vi "Location Defaults.vi"(0 "Motion Settings In":T22={"No Motion?"=FALSE, "Motion System"=enum."NI 735x", "Motion Bd ID"=1, "Motion Profile"="SMAC1", "# Axis"=1, "Reverse Z axis?"=TRUE, "SMAC Axis"=0, "scan pair"=enum."y-(x) scan", "RT fps"=6.0, "Steps per mm"=[1000, 1000, 1000, 1000], "Motor Parameters"={"velocity ct/s"=[10000.0, 10000.0, 10000.0, 50000.0], "accel ct/s^2"=[50000.0, 50000.0, 50000.0, 200000.0]}, "One Way Scan"=FALSE, "Reverse One Way Scan"=FALSE, "Global Position (mm)"=[], "Plane"=0, "Distance between\nscan lines (um)"=0.0, "Distance between\nscan planes (um)"=0.0, "number of scan planes"=1, "Total steps in line"=0, "Xtra plane\ndistance  (um)"=100, "Xtra planes "=1, "Add Axis"=FALSE, "overshoot cts"=200, "BKPT Shift"=0, "Scan Start Time (ms)"=0, "ESP VISA"="GPIB::1::INSTR", "3rd Axis"=1, "GL Ref Out"=refnum, "Galil Address"=""} {"3rd Axis" items=["x", "y", "z", "w"]; "Xtra planes" min=1; "Xtra plane\ndistance  (um)" min=0; "Distance between\nscan planes (um)" format="%.2f"; "Distance between\nscan lines (um)" format="%.2f"; "SMAC Axis" items=["None"=0, "Axis 1"=1, "Axis 2"=2, "Axis 3"=3, "Axis 4"=4, "Axis 5"=5, "Axis 6"=6, "Axis 7"=7, "Axis 8"=8, "Vector Space 1"=17, "Vector Space 2"=18, "Vector Space 3"=19, "Vector Space 4"=20]; "Motion Bd ID" min=1 max=32 step=1}, 1 "Motion System":T1=enum."No Motion Card", 2 "Debug Mode?":bool, 5 "Digitizer Settings In":T25={"Digitizer delay (us) "=0.0, "rf points per line"=2048, "lines per plane"=128, "Samp Rate (Hz)"=100000000.0, "Additional dig delay (us)"=0.0, "Voltage Scale"=0.4, "Pre-Looks"=0, "Offset delay (us)"=0.0, "bits A/D"=8, "Avg Num"=1, "DigTimeOut"=5.0, "Rel Dig Delay"=0.0, "Dig Ch"=0, "LeCroyCluster"={"LeCroy Channels"=[TRUE, FALSE, FALSE, FALSE], "LC read pt offset"=0.0, "Sweep Avg"=FALSE}, "Main Digitizer"=enum."NI Digitizer", "Dig Config"=enum."Single channel", "Digitizer ID Cluster"={"Acqiris/Alazar/SP ID"=[], "NI Instr Handles"=[], "LeCroy VISA"="", "GaGe Handle"={"Handle"=0, "Sample size"=0, "Resolution"=0, "Offset"=0, "Channels"=0, "Boards"=0}, "ATS Ref"="ATS9350", "Acqiris Address"=["PCI::INSTR0"], "ADQRef"=refnum, "adq_cu_ptr"=refnum}, "Trigger Settings"={"Trig Source"=1, "Trig Coupling"=0, "Trig Slope"=0, "Level (mV)"=1500.0}, "Bulk Acq"=FALSE, "Bulk Start Indexes"=[], "Data Ref RF"=refnum, "NI ID/Channel"=[], "Total Dig CH"=1, "Xtra Ann Trig delay (us)"=10.0, "Fix Z Delay?"=FALSE, "One Way Transmission?"=FALSE, "Data Ref Log"=refnum} {"Trigger Settings"."Trig Slope" items=["Positive", "Negative"]; "Trigger Settings"."Level (mV)" format="%.2f"; "Trigger Settings"."Trig Coupling" items=["DC 1 MOhm", "AC 1 MOhm", "DC 50 Ohm", "AC 50 Ohm"]; "Trigger Settings"."Trig Source" items=["Chan 1", "External"]; "Rel Dig Delay" format="%.2f"; "DigTimeOut" format="%.2f"; "Avg Num" min=1; "Offset delay (us)" format="%.2f"; "Additional dig delay (us)" format="%.2f"; "Digitizer delay (us)" format="%.2f"}, 6 "LeCroy IP Address":refnum<visa-resource-name>="USB0::0x05FF::0x1023::3561N17635::INSTR", 7 "Microscopy Scope":refnum<visa-resource-name>="HDO6104", 9 "Location In":T30=enum."WCM Main", 11 "Computer Name":string, 12 "Create Data Folder":bool) -> (3 "Bypass 2nd dig init":bool, 4 "Motion Settings":T22={"No Motion?"=FALSE, "Motion System"=enum."MM3000", "Motion Bd ID"=0, "Motion Profile"="SMAC1", "# Axis"=0, "Reverse Z axis?"=FALSE, "SMAC Axis"=0, "scan pair"=enum."y-(x) scan", "RT fps"=0.0, "Steps per mm"=[], "Motor Parameters"={"velocity ct/s"=[], "accel ct/s^2"=[]}, "One Way Scan"=FALSE, "Reverse One Way Scan"=FALSE, "Global Position (mm)"=[], "Plane"=0, "Distance between\nscan lines (um)"=0.0, "Distance between\nscan planes (um)"=0.0, "number of scan planes"=0, "Total steps in line"=0, "Xtra plane\ndistance  (um)"=0, "Xtra planes "=0, "Add Axis"=FALSE, "overshoot cts"=0, "BKPT Shift"=0, "Scan Start Time (ms)"=0, "ESP VISA"="", "3rd Axis"=1, "GL Ref Out"=refnum, "Galil Address"=""} {"3rd Axis" items=["x", "y", "z", "w"]; "Xtra planes" min=1; "Xtra plane\ndistance  (um)" min=0; "Distance between\nscan planes (um)" format="%.2f"; "Distance between\nscan lines (um)" format="%.2f"; "SMAC Axis" items=["None"=0, "Axis 1"=1, "Axis 2"=2, "Axis 3"=3, "Axis 4"=4, "Axis 5"=5, "Axis 6"=6, "Axis 7"=7, "Axis 8"=8, "Vector Space 1"=17, "Vector Space 2"=18, "Vector Space 3"=19, "Vector Space 4"=20]; "Motion Bd ID" min=1 max=32 step=1}, 8 "Digitizer Settings":T25={"Digitizer delay (us) "=0.0, "rf points per line"=2048, "lines per plane"=128, "Samp Rate (Hz)"=100000000.0, "Additional dig delay (us)"=0.0, "Voltage Scale"=0.4, "Pre-Looks"=0, "Offset delay (us)"=0.0, "bits A/D"=8, "Avg Num"=1, "DigTimeOut"=5.0, "Rel Dig Delay"=0.0, "Dig Ch"=0, "LeCroyCluster"={"LeCroy Channels"=[TRUE, FALSE, FALSE, FALSE], "LC read pt offset"=0.0, "Sweep Avg"=FALSE}, "Main Digitizer"=enum."NI Digitizer", "Dig Config"=enum."Single channel", "Digitizer ID Cluster"={"Acqiris/Alazar/SP ID"=[], "NI Instr Handles"=[], "LeCroy VISA"="", "GaGe Handle"={"Handle"=0, "Sample size"=0, "Resolution"=0, "Offset"=0, "Channels"=0, "Boards"=0}, "ATS Ref"="ATS9350", "Acqiris Address"=["PCI::INSTR0"], "ADQRef"=refnum, "adq_cu_ptr"=refnum}, "Trigger Settings"={"Trig Source"=1, "Trig Coupling"=0, "Trig Slope"=0, "Level (mV)"=1500.0}, "Bulk Acq"=FALSE, "Bulk Start Indexes"=[], "Data Ref RF"=refnum, "NI ID/Channel"=[], "Total Dig CH"=1, "Xtra Ann Trig delay (us)"=10.0, "Fix Z Delay?"=FALSE, "One Way Transmission?"=FALSE, "Data Ref Log"=refnum} {"Trigger Settings"."Trig Slope" items=["Positive", "Negative"]; "Trigger Settings"."Level (mV)" format="%.2f"; "Trigger Settings"."Trig Coupling" items=["DC 1 MOhm", "AC 1 MOhm", "DC 50 Ohm", "AC 50 Ohm"]; "Trigger Settings"."Trig Source" items=["Chan 1", "External"]; "Rel Dig Delay" format="%.2f"; "DigTimeOut" format="%.2f"; "Avg Num" min=1; "Offset delay (us)" format="%.2f"; "Additional dig delay (us)" format="%.2f"; "Digitizer delay (us)" format="%.2f"}, 10 "Switch T/R":u32=1, 14 "Dual XDCR Settings":T2 {"XDCR Settings"."UT340 Controls"."Low Pass Filter (MHz)" min=-6 max=60 step=1; "XDCR Settings"."UT340 Controls"."High Pass Filter (MHz)" min=1 max=20 step=1; "XDCR Settings"."UT340 Controls"."Rep Rate (Hz)" min=20 step=1; "XDCR Settings"."UT340 Controls"."Pulse Width (ns)" min=100.0 max=250.0 step=2.0; "XDCR Settings"."UT340 Controls"."Voltage" min=100 max=250 step=2; "XDCR Settings"."UT340 Controls"."PC Gain (dB)" min=2 max=72; "XDCR Settings"."UT340 Controls"."PE Gain (dB)" min=-6 max=60 step=1; "XDCR Settings"."JSR Complete"."JSR Trigger Settings"."PRF (Hz)" items=["100 Hz"=0.1, "200 Hz"=0.2, "400 Hz"=0.4, "600 Hz"=0.6, "800 Hz"=0.8, "1000 Hz"=1.0, "1250 Hz"=1.25, "1500 Hz"=1.5, "1750 Hz"=1.75, "2000 Hz"=2.0, "2500 Hz"=2.5, "3000 Hz"=3.0, "3500 Hz"=3.5, "4000 Hz"=4.0, "4500 Hz"=4.5, "5000 Hz"=5.0]; "XDCR Settings"."JSR Complete"."JSR Trigger Settings"."Trigger Source" items=["Internal", "External"]; "XDCR Settings"."JSR Complete"."JSR Trigger Settings"."External Trigger Limit" items=["No Limit", "5 kHz"]; "XDCR Settings"."JSR Complete"."JSR Receive Settings"."Gain (dB)" min=-13 max=66 step=1; "XDCR Settings"."JSR Complete"."JSR Receive Settings"."Low Pass Filter" items=["5 MHz"=5, "10 MHz"=10, "15 MHz"=15, "22.5 MHz"=22, "35 MHz"=35, "50 MHz"=50]; "XDCR Settings"."JSR Complete"."JSR Receive Settings"."High Pass Filter" items=["DC"=0, "1 MHz"=1000, "2.5 MHz"=2500, "5 MHz"=5000, "7.5 MHz"=7500, "12.5 MHz"=12500]; "XDCR Settings"."JSR Complete"."JSR Receive Settings"."Receiver Mode" items=["Echo", "Through"]; "XDCR Settings"."JSR Complete"."JSR Pulse Settings"."Pulser Voltage (V)" items=["100"=100, "125"=125, "150"=150, "175"=175, "200"=200, "225"=225, "250"=250, "275"=275, "300"=300, "325"=325, "350"=350, "375"=375, "400"=400, "425"=425, "450"=450, "475"=475]; "XDCR Settings"."JSR Complete"."JSR Pulse Settings"."Pulser Impedance" items=["High z", "Low z"]; "XDCR Settings"."JSR Complete"."JSR Pulse Settings"."Pulse Energy Level" items=["0 (Minimum)", "1", "2", "3 (Maximum)"]; "XDCR Settings"."JSR Complete"."JSR Pulse Settings"."Damping" items=["331 Ohms"=331, "198 Ohms"=198, "142 Ohms"=142, "110 Ohms"=110, "92 Ohms"=92, "77 Ohms"=77, "67 Ohms"=67, "59 Ohms"=59, "52 Ohms"=52, "47 Ohms"=47, "43 Ohms"=43, "39 Ohms"=39, "37 Ohms"=37, "34 Ohms"=34, "32 Ohms"=32, "30 Ohms"=30]; "XDCR Settings"."Panametrics Settings"."FINE ATTENUATION" items=["00.0", "00.5", "01.0", "01.5", "02.0", "02.5", "03.0", "03.5", "04.0", "04.5", "05.0", "05.5", "06.0", "06.5", "07.0", "07.5", "08.0", "08.5", "09.0", "09.5", "10.0", "10.5", "11.0", "11.5", "12.0", "12.5", "13.0", "13.5", "14.0", "14.5", "15.0", "15.5"]; "XDCR Settings"."Panametrics Settings"."COARSE ATTENUATION" items=["00.0", "10.0", "20.0", "30.0", "40.0", "50.0"]; "XDCR Settings"."Panametrics Settings"."GAIN (db)" items=["26.0", "40.0", "54.0"]; "XDCR Settings"."Panametrics Settings"."PRF (KHz)" items=["XREMT", "EXBNC", "0.200", "0.500", "1.000", "2.000", "5.000", "10.00", "20.00"]; "XDCR Settings"."Panametrics Settings"."MODE" items=["P/ E", "THRU", "RPP", "EXT_PLSR"]; "XDCR Settings"."Panametrics Settings"."LP FILT (MHz)" items=["20", "50", "100", "200"]; "XDCR Settings"."Panametrics Settings"."HP FILT (KHz)" items=["1", "1000", "3000", "10000"]; "XDCR Settings"."Panametrics Settings"."DAMPING (Ohm)" items=["7", "10", "16", "20", "26", "30", "40", "50"]; "XDCR Settings"."Panametrics Settings"."ENERGY (uJ)" items=["1", "2", "4", "8", "16", "32"]; "XDCR Settings"."Daxsonics Settings"."Freq (MHz)" items=["4"=4, "5"=5, "6"=6, "8"=8, "10"=10, "12"=12, "14"=14, "15"=15, "16"=16, "17"=17, "18"=18, "20"=20, "25"=25, "30"=30, "35"=35, "40"=40, "45"=45, "50"=50]; "XDCR Settings"."Daxsonics Settings"."Voltage (V)" items=["0"=0, "5"=5, "10"=10, "15"=15, "20"=20, "25"=25, "30"=30, "35"=35, "40"=40, "45"=45, "50"=50, "55"=55, "60"=60, "65"=65, "70"=70, "75"=75, "80"=80, "85"=85, "90"=90, "95"=95, "100"=100, "110"=110, "120"=120, "130"=130, "140"=140, "150"=150, "160"=160, "170"=170, "180"=180, "190"=190]; "XDCR Settings"."Daxsonics Settings"."Gain (dB)" items=["22"=22, "25"=25, "28"=28, "31"=31, "34"=34, "37"=37, "40"=40, "43"=43, "46"=46, "49"=49, "52"=52, "55"=55, "58"=58, "61"=61, "64"=64, "67"=67]; "XDCR Settings"."Digitizer Settings"."Additional dig delay (ms)" format="%.2f"; "XDCR Settings"."Digitizer Settings"."Time scale per Div" items=["100 ns"=0.1, "200 ns"=0.2, "500 ns"=0.5, "1 micros"=1.0, "2 micros"=2.0, "5 micros"=5.0, "10 micros"=10.0, "20 micros"=20.0, "50 micros"=50.0, "100 micros"=100.0, "200 micros"=200.0, "500 micros"=500.0, "1 ms"=1000.0, "2 ms"=2000.0, "5 ms"=5000.0, "10 ms"=10000.0, "20 ms"=20000.0, "50 ms"=50000.0, "100 ms"=100000.0, "200 ms"=200000.0]; "XDCR Settings"."Digitizer Settings"."RF data Sampling"."rf points per line" min=1; "XDCR Settings"."Digitizer Settings"."RF data Sampling"."Ref Delay (ms)" format="%.2f"}, 15 "Hardware Addresses":T29)   [LabVIEW 2022 SP3]
uses:
  Motion Controllers/NI_controller/-NI_MotionRoutines/MotionParameters.ctl
  Motion Controllers/NI_controller/-NI_MotionRoutines/MotionSys.ctl
  Motion Controllers/-MotionRoutines/ScanAxis.ctl
  Motion Controllers/-MotionRoutines/3rdAxis.ctl
  -ScanSystem/Controls/location.ctl
  Digitizers/-DigitizerRoutines/DigitizerSettings.ctl
  Digitizers/-DigitizerRoutines/Digitizer.ctl
  Digitizers/-DigitizerRoutines/DigConfig.ctl
  Digitizers/-DigitizerRoutines/DigitizerID.ctl
  C:/Windows/System32/ADQAPI_dotNet_helper.dll
  Windows/System32/ADQAPI_dotNet_helper.dll
  DualXDCR/Dual XDCR Complete Settings.ctl
  DualXDCR/XDCRSettings.ctl
  Pulsers/Daxsonics/-DaxSubroutines/Dax_Control_Cluster.ctl
  Pulsers/Panametrics/Pana5900.ctl
  Pulsers/JSR/Controls/JSR Complete.ctl
  Pulsers/JSR/Controls/JSR Pulse.ctl
  Pulsers/JSR/Controls/Damping.ctl
  Pulsers/JSR/Controls/Energy.ctl
  Pulsers/JSR/Controls/Z.ctl
  Pulsers/JSR/Controls/Volt.ctl
  Pulsers/JSR/Controls/JSR Recieve.ctl
  Pulsers/JSR/Controls/Mode.ctl
  Pulsers/JSR/Controls/HPF.ctl
  Pulsers/JSR/Controls/LPF.ctl
  Pulsers/JSR/Controls/Gain.ctl
  Pulsers/JSR/Controls/JSR Trigger.ctl
  Pulsers/JSR/Controls/Trig Limit.ctl
  Pulsers/JSR/Controls/Trig Source.ctl
  Pulsers/JSR/Controls/PRF.ctl
  Pulsers/UTEX/Controls/UTEX Controls.ctl
  Motion Controllers/-MotionRoutines/MotionGlobals.vi
  Pulsers/PulserGlobals.vi
  Switch Modules/SwitchGlobals.vi
panel:
  in  "Microscopy Scope 2":refnum<visa-resource-name>="HDO6104"
  # "1-D and 2-D B scan settings"
  # "1-D and 2-D B scan settings"
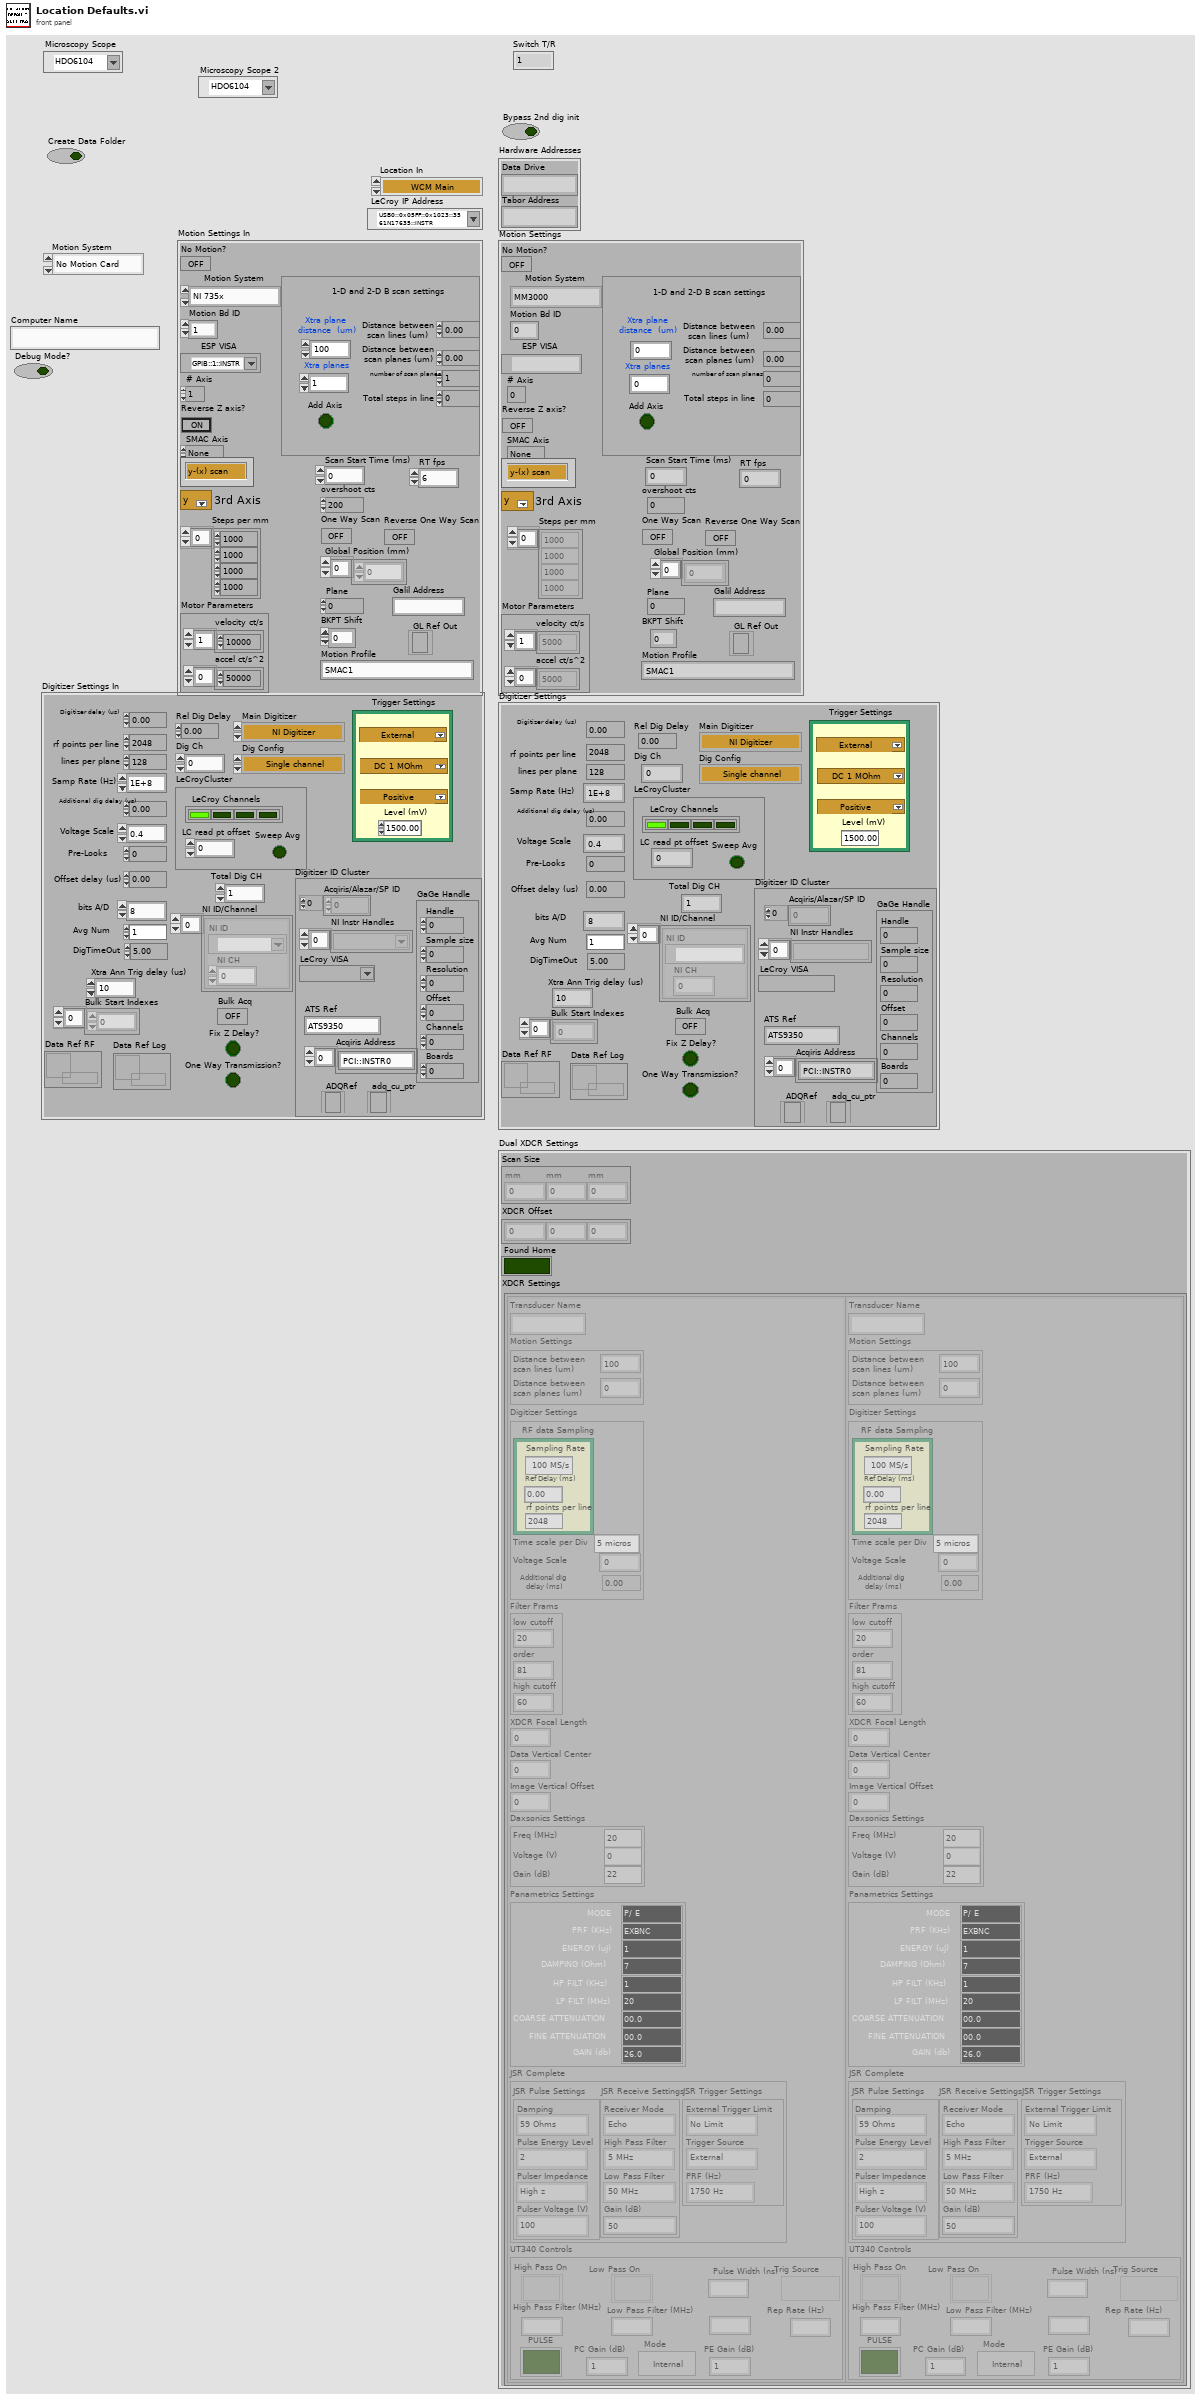
[diagram p1: front panel]
types:
  T1 = typedef "MotionSys.ctl" = enum16{"MM3000", "NI 735x", "Newport ESP", "No Motion Card", "Galil"}
  T2 = typedef "Dual XDCR Complete Settings.ctl" = cluster{"Scan Size":dbl[], "XDCR Offset":dbl[], "Found Home":bool, "XDCR Settings":T3[]}
  T3 = typedef "XDCRSettings.ctl" = cluster{"Transducer Name":string, "Motion Settings":cluster{"Distance between\nscan lines (um)":sgl, "Distance between\nscan planes (um)":sgl}, "Digitizer Settings":cluster{"RF data Sampling":cluster{"Sampling Rate":dbl, "Ref Delay (ms)":dbl, "rf points per line":i32}, "Time scale per Div":dbl, "Voltage Scale":dbl, "Additional dig delay (ms)":dbl}, "Filter Prams":cluster{"low cutoff":i32, "order":i32, "high cutoff":i32}, "XDCR Focal Length":dbl, "Data Vertical Center":dbl, "Image Vertical Offset":dbl, "Daxsonics Settings":T4, "Panametrics Settings":T5, "JSR Complete":T6, "UT340 Controls":T21}
  T4 = typedef "Dax_Control_Cluster.ctl" = cluster{"Freq (MHz) ":u16, "Voltage (V)":u16, "Gain (dB)":u16}
  T5 = typedef "Pana5900.ctl" = cluster{"ENERGY (uJ)":u16, "DAMPING (Ohm)":u16, "HP FILT (KHz) ":u16, "LP FILT (MHz)":u16, "MODE":u16, "PRF (KHz)":u16, "GAIN (db)":u16, "COARSE ATTENUATION":u16, "FINE ATTENUATION":u16}
  T6 = typedef "JSR Complete.ctl" = cluster{"JSR Pulse Settings":T7, "JSR Receive Settings":T12, "JSR Trigger Settings":T17}
  T7 = typedef "JSR Pulse.ctl" = cluster{"Damping":T8, "Pulse Energy Level":T9, "Pulser Impedance":T10, "Pulser Voltage (V)":T11}
  T8 = typedef "Damping.ctl" = i16
  T9 = typedef "Energy.ctl" = u16
  T10 = typedef "Z.ctl" = u16
  T11 = typedef "Volt.ctl" = i16
  T12 = typedef "JSR Recieve.ctl" = cluster{"Receiver Mode":T13, "High Pass Filter":T14, "Low Pass Filter":T15, "Gain (dB)":T16}
  T13 = typedef "Mode.ctl" = i8
  T14 = typedef "HPF.ctl" = u16
  T15 = typedef "LPF.ctl" = u16
  T16 = typedef "Gain.ctl" = i8
  T17 = typedef "JSR Trigger.ctl" = cluster{"External Trigger Limit":T18, "Trigger Source":T19, "PRF (Hz)":T20}
  T18 = typedef "Trig Limit.ctl" = i8
  T19 = typedef "Trig Source.ctl" = i8
  T20 = typedef "PRF.ctl" = dbl
  T21 = typedef "UTEX Controls.ctl" = cluster{"High Pass On":bool, "High Pass Filter (MHz)":i16, "Low Pass On":bool, "Low Pass Filter (MHz)":i16, "PE Gain (dB)":i16, "Voltage":i16, "Pulse Width (ns)":dbl, "Mode":bool, "PC Gain (dB)":i16, "Trig Source":bool, "Rep Rate (Hz)":i16, "PULSE":bool}
  T22 = typedef "MotionParameters.ctl" = cluster{"No Motion?":bool, "Motion System":T1, "Motion Bd ID":u8, "Motion Profile":string, "# Axis":i8, "Reverse Z axis?":bool, "SMAC Axis":u16, "scan pair":T23, "RT fps":sgl, "Steps per mm":i32[], "Motor Parameters":cluster{"velocity ct/s":dbl[], "accel ct/s^2":dbl[]}, "One Way Scan":bool, "Reverse One Way Scan":bool, "Global Position (mm)":dbl[], "Plane":i32, "Distance between\nscan lines (um)":sgl, "Distance between\nscan planes (um)":sgl, "number of scan planes":i32, "Total steps in line":i32, "Xtra plane\ndistance  (um)":i32, "Xtra planes ":i32, "Add Axis":bool, "overshoot cts":i32, "BKPT Shift":i32, "Scan Start Time (ms)":u32, "ESP VISA":refnum<visa-resource-name>, "3rd Axis":T24, "GL Ref Out":refnum<k7>, "Galil Address":string}
  T23 = typedef "ScanAxis.ctl" = enum16{"y-(x) scan", "x-(y) scan", "z-(x) scan", "z-(y) scan", "y-(z) scan", "x-(z) scan", "w-(x) scan", "w-(y) scan", "w-(z) scan", "x-(w) scan", "y-(w) scan", "z-(w) scan"}
  T24 = typedef "3rdAxis.ctl" = u16
  T25 = typedef "DigitizerSettings.ctl" = cluster{"Digitizer delay (us) ":dbl, "rf points per line":i32, "lines per plane":i32, "Samp Rate (Hz)":dbl, "Additional dig delay (us)":dbl, "Voltage Scale":dbl, "Pre-Looks":i32, "Offset delay (us)":dbl, "bits A/D":i8, "Avg Num":i32, "DigTimeOut":sgl, "Rel Dig Delay":sgl, "Dig Ch":i32, "LeCroyCluster":cluster{"LeCroy Channels":bool[], "LC read pt offset":dbl, "Sweep Avg":bool}, "Main Digitizer":T26, "Dig Config":T27, "Digitizer ID Cluster":T28, "Trigger Settings":cluster{"Trig Source":u16, "Trig Coupling":u16, "Trig Slope":u16, "Level (mV)":dbl}, "Bulk Acq":bool, "Bulk Start Indexes":i32[], "Data Ref RF":refnum<data-value>, "NI ID/Channel":cluster{"NI ID":refnum<k15>, "NI CH":i32}[], "Total Dig CH":i32, "Xtra Ann Trig delay (us)":dbl, "Fix Z Delay?":bool, "One Way Transmission?":bool, "Data Ref Log":refnum<data-value>}
  T26 = typedef "Digitizer.ctl" = enum16{"Acqiris Digitizer", "NI Digitizer", "LeCroy", "GaGe", "AlazarTech", "No Digitizer", "Teledyne"}
  T27 = typedef "DigConfig.ctl" = enum16{"Single channel", "2 Chans w/ 2 Acqiris", "2 Chans w/ 1 Acqiris", "5-CH Pulser New", "5-CH pulser w/ ann array", "5-pass style ann array", "Empty"}
  T28 = typedef "DigitizerID.ctl" = cluster{"Acqiris/Alazar/SP ID":u32[], "NI Instr Handles":refnum<k15>[], "LeCroy VISA":refnum<visa-resource-name>, "GaGe Handle":cluster{"Handle":u32, "Sample size":u32, "Resolution":i32, "Offset":i32, "Channels":u32, "Boards":u32}, "ATS Ref":string, "Acqiris Address":string[], "ADQRef":refnum<k24>, "adq_cu_ptr":refnum<k24>}
  T29 = cluster{"Data Drive":string, "Tabor Address":string}
  T30 = typedef "location.ctl" = enum16{"Automatic", "WCM Main", "Hawaii", "Columbia MM3000", "Columbia  NI System", "NYU", "RRI 2", "UHI Allen", "CUMC RT", "Chiba", "Stony Brook", "WCM Microscopy", "WCM Aeoretch", "WCM Optics Lab", "WCM Main 2Axis", "WCM Rotation", "WCM SAM SMAC", "SERI GP", "SERI SAM 2023"}
  T31 = cluster{"velocity mm/s":dbl[], "accel mm/s^2":dbl[]}
  T32 = cluster{"velocity\nmm/s":dbl[], "accel\nmm/s^2":dbl[]}
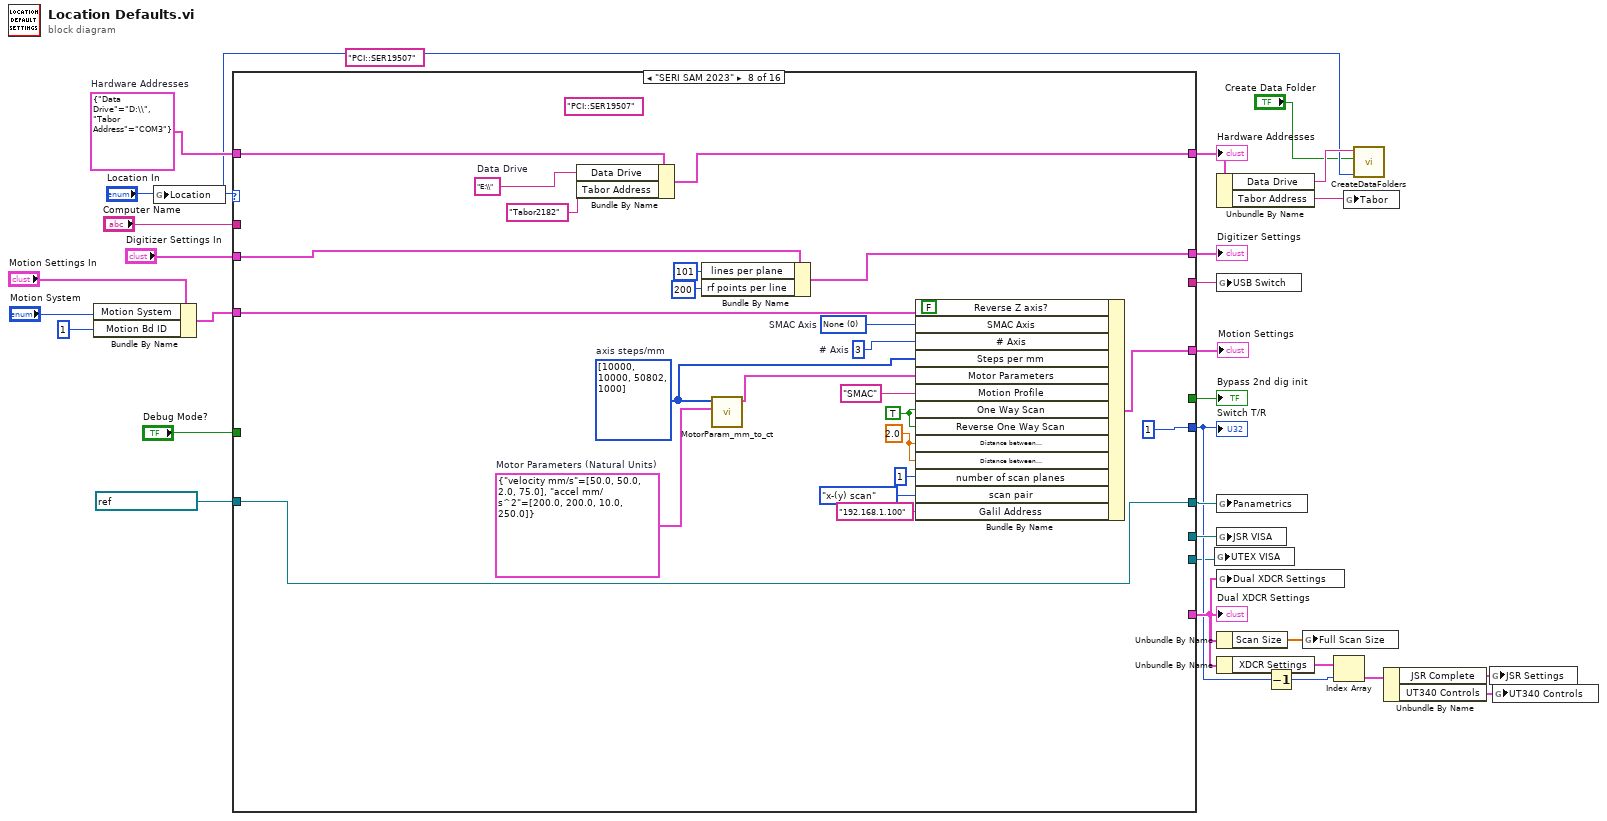
[diagram p0: block diagram]
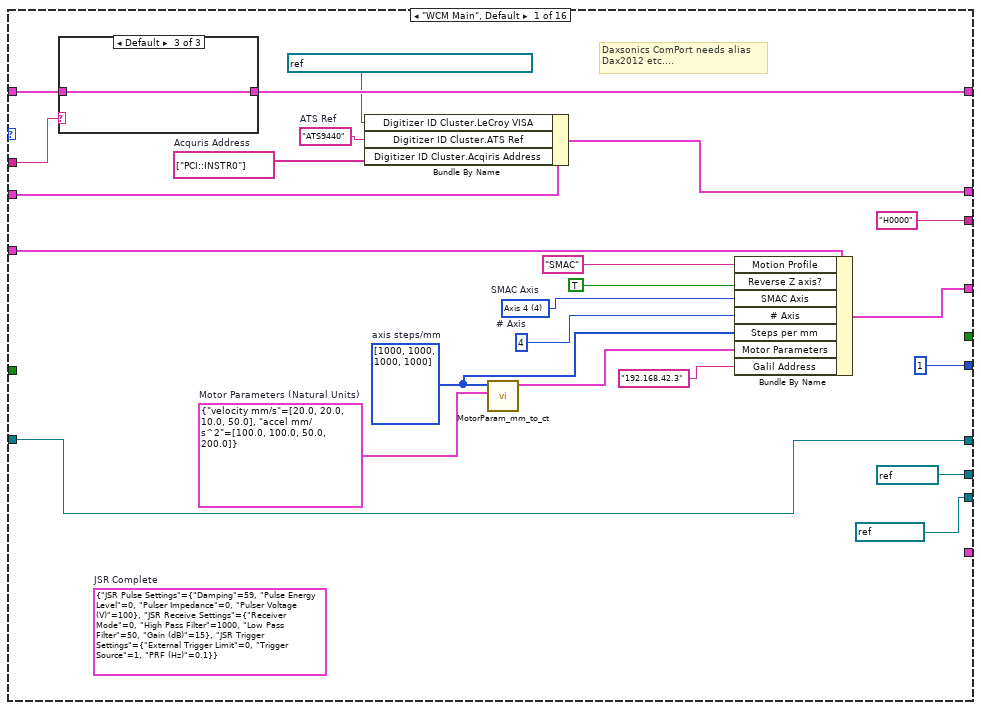
[diagram p2: hidden frame]
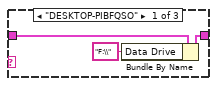
[diagram p3: hidden frame]
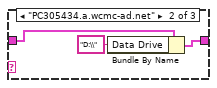
[diagram p4: hidden frame]
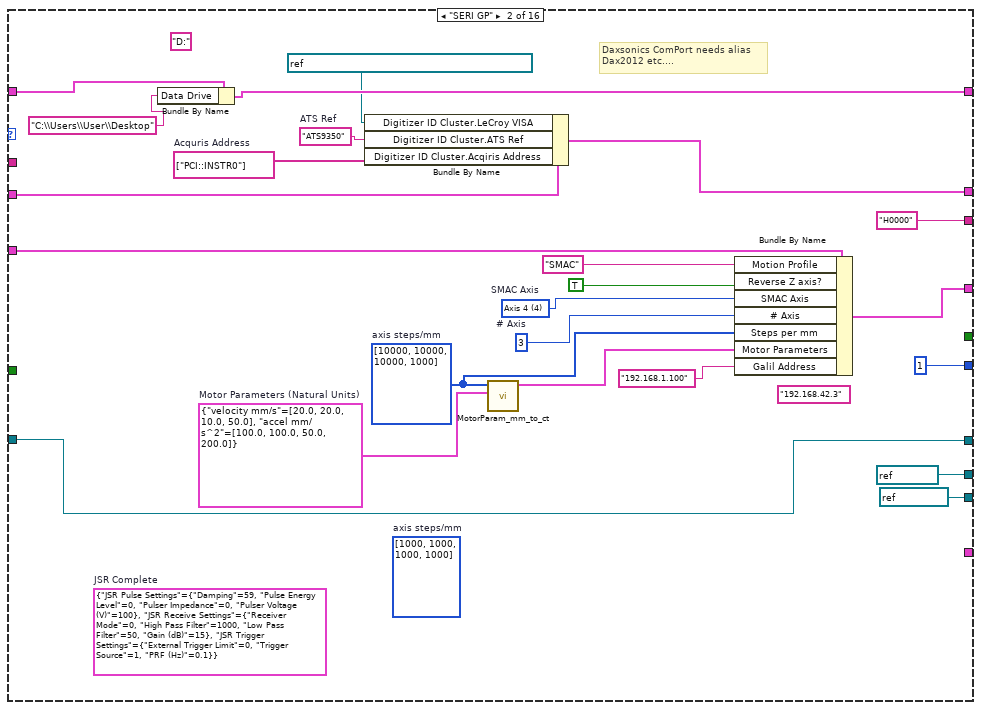
[diagram p5: hidden frame]
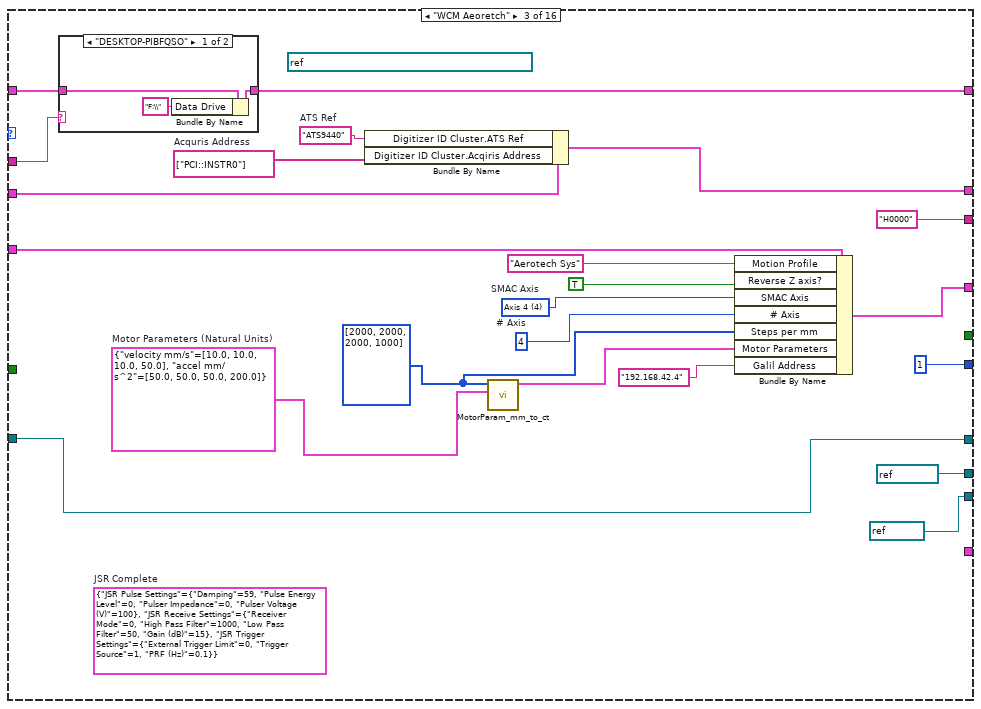
[diagram p6: hidden frame]
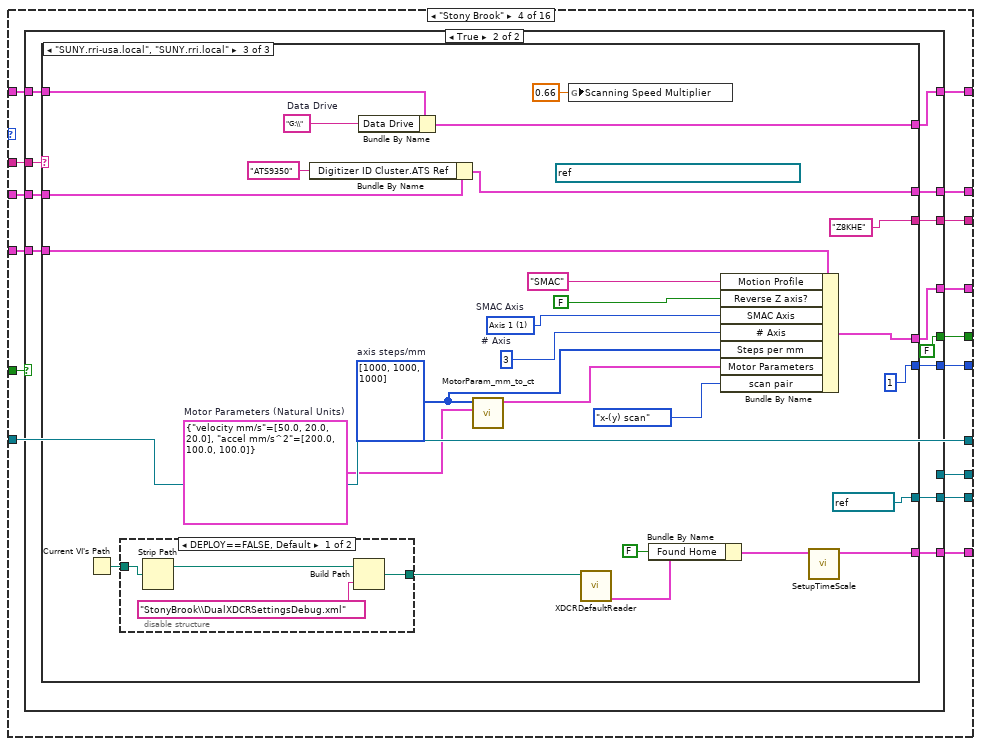
[diagram p8: hidden frame]
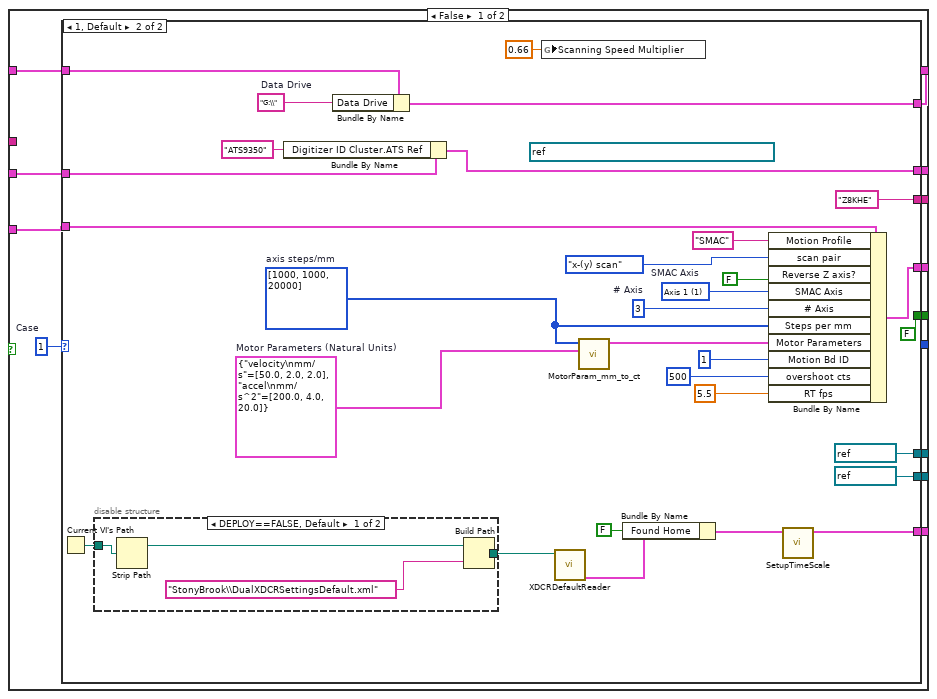
[diagram p9: hidden frame]
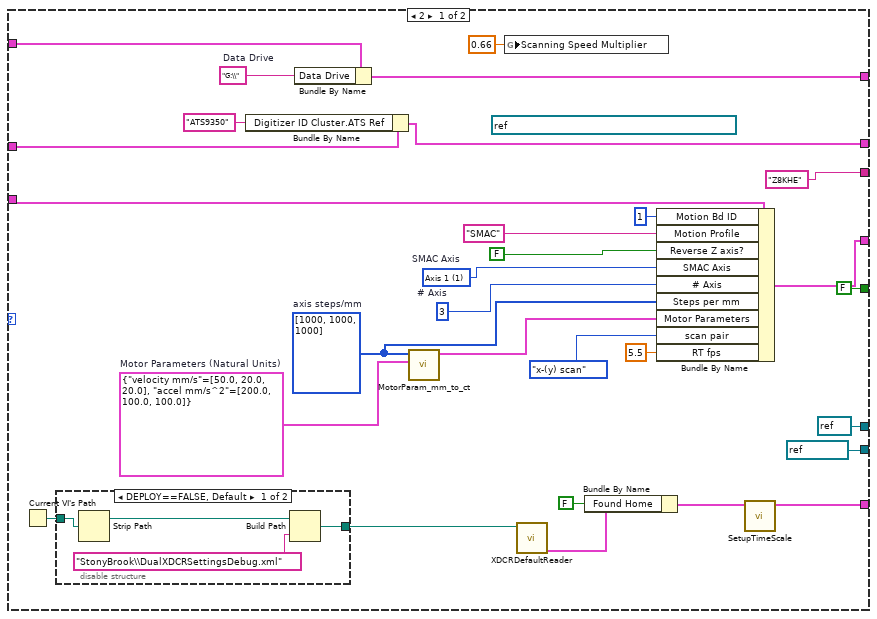
[diagram p10: hidden frame]
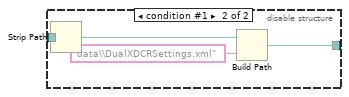
[diagram p11: hidden frame]
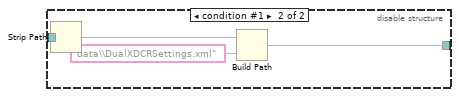
[diagram p12: hidden frame]
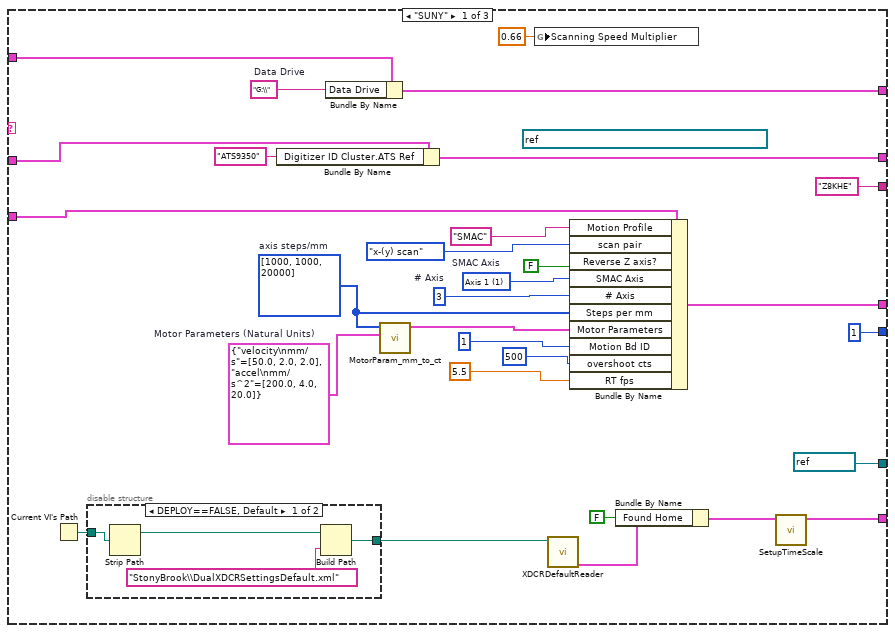
[diagram p13: hidden frame]
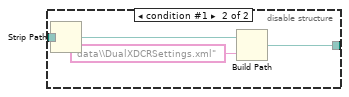
[diagram p14: hidden frame]
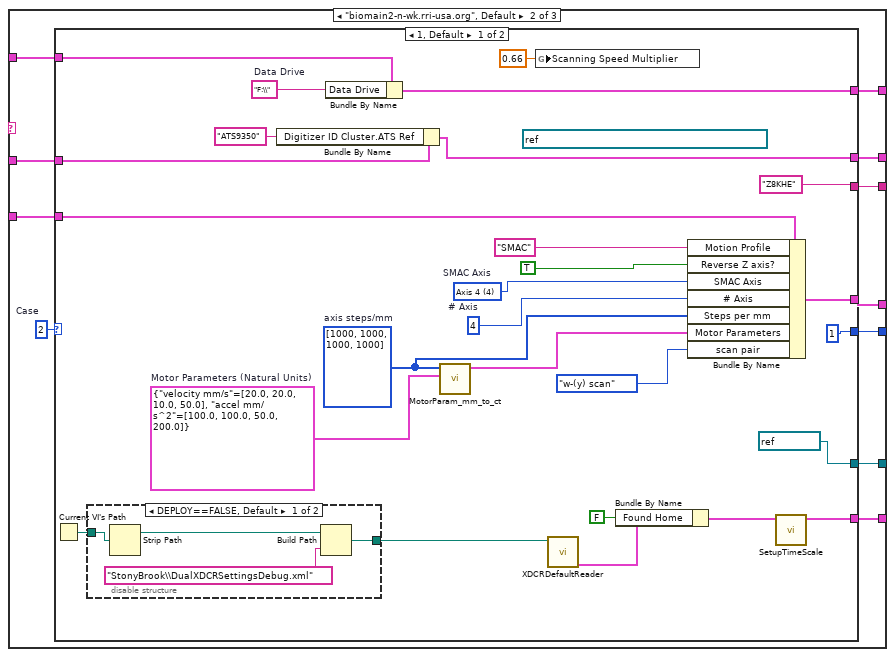
[diagram p15: hidden frame]
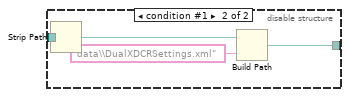
[diagram p16: hidden frame]
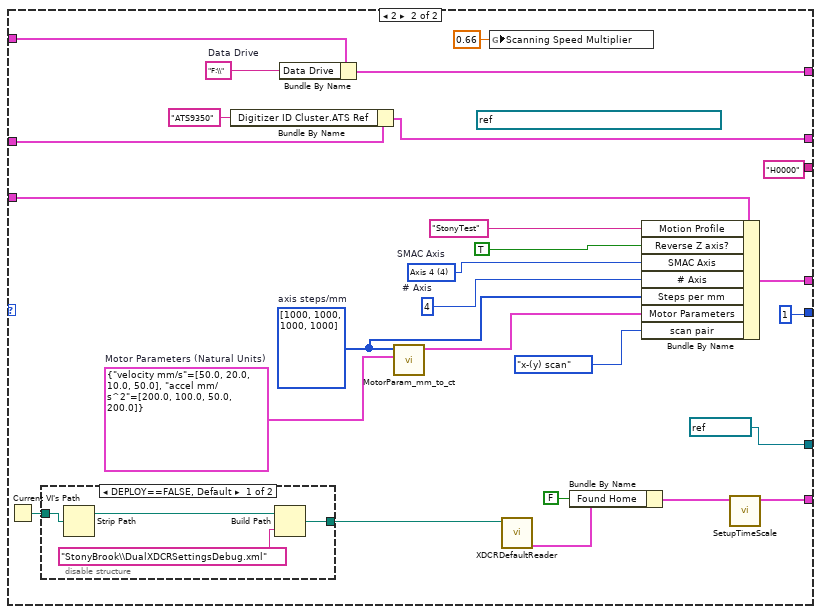
[diagram p17: hidden frame]
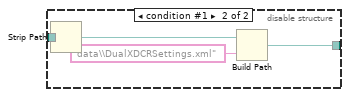
[diagram p18: hidden frame]
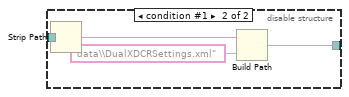
[diagram p19: hidden frame]
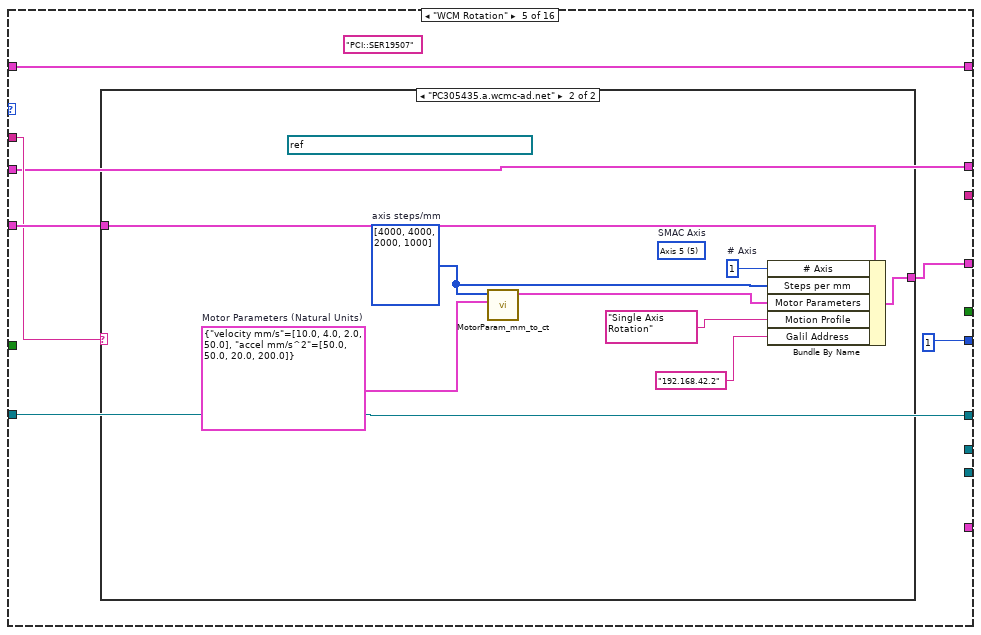
[diagram p20: hidden frame]
diagram:
  (unwired) "PCI::SER19507" ("ResourceName")
  w28 = T29 {"Data Drive"="D:\\", "Tabor Address"="COM3"}  # Hardware Addresses
  n1 = Bundle By Name(cluster="Motion Settings In", "Motion System"="Motion System", "Motion Bd ID"=u8 1 ("Board ID")) -> (w19:T22)
  n2 = global write "MotionGlobals.vi" "Location"("Location In") -> ()
  n3 = case shown="\"SERI SAM 2023\"" "Location In" {
    tunnel: [_ _ _ w118 _ _ _ _ _ _ _ TRUE TRUE _ TRUE _] -> w29
    tunnel: [w52 w82 w104 w123 w379 w418 w442 w466 w476 w490 w498 w655 w675 w700 w716 w738] -> w23
    tunnel: w19 -> [w51 w81 w103 w119 w378 w417 w441 w465 w470 w489 w503 w654 w674 w699 w715 w730]
    tunnel: [w41 w72 w95 w120 w373 w401 w425 w450 w473 w485 w499 w645 w665 w689 w709 w727] -> w22
    tunnel: "Digitizer Settings In" -> [w42 w73 w96 w121 w373 w408 w432 w456 w473 w485 w500 w646 w666 w692 w709 w729]
    tunnel: w28 -> [w38 w69 w92 w122 w377 w411 w435 w459 w472 w483 w502 w650 w670 w693 w711 w731]
    tunnel: [w37 w68 w91 w117 w377 w410 w434 w458 w472 w483 w501 w649 w669 w694 w710 w732] -> w27
    tunnel: [_ _ _ w116 _ _ _ _ _ _ w497 _ _ _ _ _] -> w8
    tunnel: [u32 1 ("Switch T/R") u32 1 ("Switch T/R") u32 1 ("Switch T/R") w109 u32 1 ("Switch T/R") u32 1 ("Switch T/R") u32 1 ("Switch T/R") u32 1 ("Switch T/R") u32 1 ("Switch T/R") u32 1 ("Switch T/R") _ _ _ u32 1 ("Switch T/R") _ _] -> w4
    tunnel: "Computer Name" -> [w36 _ w90 w112 w374 _ _ _ _ _ w493 _ _ _ _ _]
    tunnel: ["H0000" "H0000" "H0000" w115 _ _ _ _ _ _ w496 _ _ _ _ _] -> w14
    tunnel: [w34 w66 w88 w114 w375 w397 w421 w446 w468 w481 w495 refnum<visa-resource-name> "GPIB0::9::INSTR" ("VISA resource name") w658 w680 w708 w725] -> w13
    tunnel: refnum<visa-resource-name> "GPIB::1::INSTR" ("VISA resource name") -> [w34 w66 w88 w114 w375 w397 w421 w446 w468 w481 _ _ w658 w680 w708 w725]
    tunnel: "Debug Mode?" -> [_ _ _ w113 _ _ _ _ _ _ w494 _ _ _ _ _]
    tunnel: [refnum<visa-resource-name> "COM4" ("JSR VISA") refnum<visa-resource-name> "COM4" ("JSR VISA") refnum<visa-resource-name> "COM4" ("JSR VISA") w111 _ _ _ _ _ _ _ _ _ _ _ _] -> w9
    tunnel: [refnum<visa-resource-name> "UTEX" ("JSR VISA") refnum<visa-resource-name> "UTEX" ("JSR VISA") refnum<visa-resource-name> "UTEX" ("JSR VISA") w110 _ _ _ _ _ _ _ _ _ _ _ _] -> w2
    frame "WCM Main", Default {
      (unwired) T6 {"JSR Pulse Settings"={"Damping"=59, "Pulse Energy Level"=0, "Pulser Impedance"=0, "Pulser Voltage (V)"=100}, "JSR Receive Settings"={"Receiver Mode"=0, "High Pass Filter"=1000, "Low Pass Filter"=50, "Gain (dB)"=15}, "JSR Trigger Settings"={"External Trigger Limit"=0, "Trigger Source"=1, "PRF (Hz)"=0.1}}  # JSR Complete
      w40 = "ATS9440"  # ATS Ref
      w39 = string[] ["PCI::INSTR0"]  # Acquris Address
      w47 = i32[] [1000, 1000, 1000, 1000]  # axis steps/mm
      w46 = T31 {"velocity mm/s"=[20.0, 20.0, 10.0, 50.0], "accel mm/s^2"=[100.0, 100.0, 50.0, 200.0]}  # Motor Parameters (Natural Units)
      w48 = i8 4  # # Axis
      w49 = u16 4 items=["None"=0, "Axis 1"=1, "Axis 2"=2, "Axis 3"=3, "Axis 4"=4, "Axis 5"=5, "Axis 6"=6, "Axis 7"=7, "Axis 8"=8, "Vector Space 1"=17, "Vector Space 2"=18, "Vector Space 3"=19, "Vector Space 4"=20]  # SMAC Axis
      # "Daxsonics ComPort needs alias\nDax2012 etc...."
      n4 = case shown="Default" w36 {
        tunnel: w38 -> [w55 w57 w59]
        tunnel: [w54 w56 w59] -> w37
        frame "DESKTOP-PIBFQSO" {
          n5 = Bundle By Name(cluster=w55, "Data Drive"="F:\\") -> (w54:T29)
        }
        frame "PC305434.a.wcmc-ad.net" {
          n6 = Bundle By Name(cluster=w57, "Data Drive"="D:\\") -> (w56:T29)
        }
        frame Default {
        }
      }
      n7 = Bundle By Name(cluster=w42, "Digitizer ID Cluster.LeCroy VISA"=refnum<visa-resource-name> "USB0::0x05FF::0x1023::3504N04910::INSTR" ("VISA resource name"), "Digitizer ID Cluster.ATS Ref"=w40, "Digitizer ID Cluster.Acqiris Address"=w39) -> (w41:T25)
      n8 = call "MotorParam_mm_to_ct.vi"("Motor Parameters (Natural Units)"=w46, "Counts / mm"=w47) -> ("Motoar Parameters (counts)"=w45:cluster{dbl[], dbl[]})  [unwired: 9 in]
      n9 = Bundle By Name(cluster=w51, "Motion Profile"="SMAC", "Reverse Z axis?"=TRUE, "SMAC Axis"=w49, "# Axis"=w48, "Steps per mm"=w47, "Motor Parameters"=w45, "Galil Address"="192.168.42.3" ("For Galil")) -> (w52:T22)
    }
    frame "SERI GP" {
      (unwired) i32[] [1000, 1000, 1000, 1000]  # axis steps/mm
      (unwired) "D:" ("Data Drive")
      (unwired) "192.168.42.3" ("For Galil")
      (unwired) T6 {"JSR Pulse Settings"={"Damping"=59, "Pulse Energy Level"=0, "Pulser Impedance"=0, "Pulser Voltage (V)"=100}, "JSR Receive Settings"={"Receiver Mode"=0, "High Pass Filter"=1000, "Low Pass Filter"=50, "Gain (dB)"=15}, "JSR Trigger Settings"={"External Trigger Limit"=0, "Trigger Source"=1, "PRF (Hz)"=0.1}}  # JSR Complete
      w71 = "ATS9350"  # ATS Ref
      w70 = string[] ["PCI::INSTR0"]  # Acquris Address
      w61 = i32[] [10000, 10000, 10000, 1000]  # axis steps/mm
      w77 = T31 {"velocity mm/s"=[20.0, 20.0, 10.0, 50.0], "accel mm/s^2"=[100.0, 100.0, 50.0, 200.0]}  # Motor Parameters (Natural Units)
      w78 = i8 3  # # Axis
      w79 = u16 4 items=["None"=0, "Axis 1"=1, "Axis 2"=2, "Axis 3"=3, "Axis 4"=4, "Axis 5"=5, "Axis 6"=6, "Axis 7"=7, "Axis 8"=8, "Vector Space 1"=17, "Vector Space 2"=18, "Vector Space 3"=19, "Vector Space 4"=20]  # SMAC Axis
      # "Daxsonics ComPort needs alias\nDax2012 etc...."
      n10 = Bundle By Name(cluster=w69, "Data Drive"="C:\\Users\\User\\Desktop") -> (w68:T29)
      n11 = Bundle By Name(cluster=w73, "Digitizer ID Cluster.LeCroy VISA"=refnum<visa-resource-name> "USB0::0x05FF::0x1023::3504N04910::INSTR" ("VISA resource name"), "Digitizer ID Cluster.ATS Ref"=w71, "Digitizer ID Cluster.Acqiris Address"=w70) -> (w72:T25)
      n12 = call "MotorParam_mm_to_ct.vi"("Motor Parameters (Natural Units)"=w77, "Counts / mm"=w61) -> ("Motoar Parameters (counts)"=w76:cluster{dbl[], dbl[]})  [unwired: 9 in]
      n13 = Bundle By Name(cluster=w81, "Motion Profile"="SMAC", "Reverse Z axis?"=TRUE, "SMAC Axis"=w79, "# Axis"=w78, "Steps per mm"=w61, "Motor Parameters"=w76, "Galil Address"="192.168.1.100" ("For Galil")) -> (w82:T22)
    }
    frame "WCM Aeoretch" {
      w84 = T31 {"velocity mm/s"=[10.0, 10.0, 10.0, 50.0], "accel mm/s^2"=[50.0, 50.0, 50.0, 200.0]}  # Motor Parameters (Natural Units)
      w83 = i32[] [2000, 2000, 2000, 1000]
      (unwired) T6 {"JSR Pulse Settings"={"Damping"=59, "Pulse Energy Level"=0, "Pulser Impedance"=0, "Pulser Voltage (V)"=100}, "JSR Receive Settings"={"Receiver Mode"=0, "High Pass Filter"=1000, "Low Pass Filter"=50, "Gain (dB)"=15}, "JSR Trigger Settings"={"External Trigger Limit"=0, "Trigger Source"=1, "PRF (Hz)"=0.1}}  # JSR Complete
      w94 = "ATS9440"  # ATS Ref
      w93 = string[] ["PCI::INSTR0"]  # Acquris Address
      (unwired) refnum<visa-resource-name> "USB0::0x05FF::0x1023::3504N04910::INSTR" ("VISA resource name")
      w100 = i8 4  # # Axis
      w101 = u16 4 items=["None"=0, "Axis 1"=1, "Axis 2"=2, "Axis 3"=3, "Axis 4"=4, "Axis 5"=5, "Axis 6"=6, "Axis 7"=7, "Axis 8"=8, "Vector Space 1"=17, "Vector Space 2"=18, "Vector Space 3"=19, "Vector Space 4"=20]  # SMAC Axis
      n14 = case shown="\"DESKTOP-PIBFQSO\"" w90 {
        tunnel: w92 -> [w107 w108]
        tunnel: [w106 w108] -> w91
        frame "DESKTOP-PIBFQSO" {
          n15 = Bundle By Name(cluster=w107, "Data Drive"="F:\\") -> (w106:T29)
        }
        frame Default {
        }
      }
      n16 = Bundle By Name(cluster=w96, "Digitizer ID Cluster.ATS Ref"=w94, "Digitizer ID Cluster.Acqiris Address"=w93) -> (w95:T25)
      n17 = call "MotorParam_mm_to_ct.vi"("Motor Parameters (Natural Units)"=w84, "Counts / mm"=w83) -> ("Motoar Parameters (counts)"=w99:cluster{dbl[], dbl[]})  [unwired: 9 in]
      n18 = Bundle By Name(cluster=w103, "Motion Profile"="Aerotech Sys", "Reverse Z axis?"=TRUE, "SMAC Axis"=w101, "# Axis"=w100, "Steps per mm"=w83, "Motor Parameters"=w99, "Galil Address"="192.168.42.4" ("For Galil")) -> (w104:T22)
    }
    frame "Stony Brook" {
      n19 = case shown="True" w113 {
        tunnel: [w135 w218] -> w123
        tunnel: w122 -> [w134 w221]
        tunnel: w121 -> [w133 w215]
        tunnel: [w132 w216] -> w120
        tunnel: w119 -> [w131 w219]
        tunnel: [w130 FALSE] -> w118
        tunnel: [w129 w220] -> w117
        tunnel: [w128 w214] -> w116
        tunnel: [w127 w217] -> w115
        tunnel: w112 -> [_ w222]
        tunnel: [w125 _] -> w111
        tunnel: [w124 w212] -> w110
        tunnel: [_ w211] -> w109
        frame False {
          w126 = i8 1  # Case
          n20 = case shown="1, Default" w126 {
            tunnel: [w145 w202] -> w135
            tunnel: w134 -> [w141 w196]
            tunnel: w133 -> [w142 w195]
            tunnel: [w147 w190] -> w132
            tunnel: w131 -> [w140 w188]
            tunnel: [FALSE FALSE] -> w130
            tunnel: [w146 w185] -> w129
            tunnel: [w143 w180] -> w128
            tunnel: ["Z8KHE" "Z8KHE"] -> w127
            tunnel: [refnum<visa-resource-name> refnum ("JSR VISA") refnum<visa-resource-name> "COM7" ("JSR VISA")] -> w125
            tunnel: [refnum<visa-resource-name> "COM4" ("JSR VISA") refnum<visa-resource-name> "COM7" ("JSR VISA")] -> w124
            frame 2 {
              w153 = i32[] [1000, 1000, 1000]  # axis steps/mm
              w152 = T31 {"velocity mm/s"=[50.0, 20.0, 20.0], "accel mm/s^2"=[200.0, 100.0, 100.0]}  # Motor Parameters (Natural Units)
              w154 = i8 3  # # Axis
              w155 = u16 1 items=["None"=0, "Axis 1"=1, "Axis 2"=2, "Axis 3"=3, "Axis 4"=4, "Axis 5"=5, "Axis 6"=6, "Axis 7"=7, "Axis 8"=8, "Vector Space 1"=17, "Vector Space 2"=18, "Vector Space 3"=19, "Vector Space 4"=20]  # SMAC Axis
              w163 = "G:\\"  # Data Drive
              (unwired) refnum<visa-resource-name> "USB0::0x05FF::0x1023::3504N04910::INSTR" ("VISA resource name")
              n21 = Current VI's Path() -> (path=w159:path)
              n22 = disable-structure shown="DEPLOY==FALSE, Default" {
                disable-tunnel: w159 -> [w168 w172]
                disable-tunnel: [w165 w170] -> w158
                frame condition #0 (active) {
                  n23 = Strip Path(path=w168) -> (stripped path=w166:path)  [unwired: 1 out]
                  n24 = Build Path(base path=w166, name or relative path="StonyBrook\\DualXDCRSettingsDebug.xml") -> (appended path=w165:path)
                }
                frame condition #1 {
                  n25 = Strip Path(path=w172) -> (stripped path=w169:path)  [unwired: 1 out]
                  n26 = Build Path(base path=w169, name or relative path="data\\DualXDCRSettings.xml") -> (appended path=w170:path)
                }
              }
              n27 = Bundle By Name(cluster=w142, "Digitizer ID Cluster.ATS Ref"="ATS9350") -> (w147:T25)
              n28 = Bundle By Name(cluster=w141, "Data Drive"=w163) -> (w146:T29)
              n29 = call "MotorParam_mm_to_ct.vi"("Motor Parameters (Natural Units)"=w152, "Counts / mm"=w153) -> ("Motoar Parameters (counts)"=w151:cluster{dbl[], dbl[]})  [unwired: 9 in]
              n30 = global write "MotionGlobals.vi" "Scanning Speed Multiplier"(0.66 ("Scanning Speed Multiplier")) -> ()
              n31 = call "XDCRDefaultReader.vi"("path to XML document"=w158) -> ("Dual XDCR Settings"=w161:T2)  [unwired: 10 in]
              n32 = Bundle By Name(cluster=w161, "Found Home"=FALSE) -> (w160:T2)
              n33 = Bundle By Name(cluster=w140, "Motion Bd ID"=u8 1 ("Board ID"), "Motion Profile"="SMAC", "Reverse Z axis?"=FALSE, "SMAC Axis"=w155, "# Axis"=w154, "Steps per mm"=w153, "Motor Parameters"=w151, "scan pair"=ScanAxis."x-(y) scan", "RT fps"=sgl 5.5) -> (w145:T22)
              n34 = call "SetupTimeScale.vi"("Dual XDCR Settings in"=w160) -> ("Dual XDCR Settings out"=w143:T2)  [unwired: 10 in]
            }
            frame 1, Default {
              w184 = "G:\\"  # Data Drive
              w192 = T32 {"velocity\nmm/s"=[50.0, 2.0, 2.0], "accel\nmm/s^2"=[200.0, 4.0, 20.0]}  # Motor Parameters (Natural Units)
              w191 = i32[] [1000, 1000, 20000]  # axis steps/mm
              (unwired) refnum<visa-resource-name> "USB0::0x05FF::0x1023::3504N04910::INSTR" ("VISA resource name")
              w199 = i8 3  # # Axis
              w200 = u16 1 items=["None"=0, "Axis 1"=1, "Axis 2"=2, "Axis 3"=3, "Axis 4"=4, "Axis 5"=5, "Axis 6"=6, "Axis 7"=7, "Axis 8"=8, "Vector Space 1"=17, "Vector Space 2"=18, "Vector Space 3"=19, "Vector Space 4"=20]  # SMAC Axis
              n35 = Current VI's Path() -> (path=w178:path)
              n36 = disable-structure shown="DEPLOY==FALSE, Default" {
                disable-tunnel: w178 -> [w206 w210]
                disable-tunnel: [w204 w208] -> w177
                frame condition #0 (active) {
                  n37 = Strip Path(path=w206) -> (stripped path=w205:path)  [unwired: 1 out]
                  n38 = Build Path(base path=w205, name or relative path="StonyBrook\\DualXDCRSettingsDefault.xml") -> (appended path=w204:path)
                }
                frame condition #1 {
                  n39 = Strip Path(path=w210) -> (stripped path=w207:path)  [unwired: 1 out]
                  n40 = Build Path(base path=w207, name or relative path="data\\DualXDCRSettings.xml") -> (appended path=w208:path)
                }
              }
              n41 = Bundle By Name(cluster=w195, "Digitizer ID Cluster.ATS Ref"="ATS9350") -> (w190:T25)
              n42 = Bundle By Name(cluster=w196, "Data Drive"=w184) -> (w185:T29)
              n43 = global write "MotionGlobals.vi" "Scanning Speed Multiplier"(0.66 ("Scanning Speed Multiplier")) -> ()
              n44 = call "XDCRDefaultReader.vi"("path to XML document"=w177) -> ("Dual XDCR Settings"=w182:T2)  [unwired: 10 in]
              n45 = call "MotorParam_mm_to_ct.vi"("Motor Parameters (Natural Units)"=w192, "Counts / mm"=w191) -> ("Motoar Parameters (counts)"=w198:cluster{dbl[], dbl[]})  [unwired: 9 in]
              n46 = Bundle By Name(cluster=w182, "Found Home"=FALSE) -> (w181:T2)
              n47 = Bundle By Name(cluster=w188, "Motion Profile"="SMAC", "scan pair"=ScanAxis."x-(y) scan", "Reverse Z axis?"=FALSE, "SMAC Axis"=w200, "# Axis"=w199, "Steps per mm"=w191, "Motor Parameters"=w198, "Motion Bd ID"=u8 1 ("Board ID"), "overshoot cts"=500, "RT fps"=sgl 5.5) -> (w202:T22)
              n48 = call "SetupTimeScale.vi"("Dual XDCR Settings in"=w181) -> ("Dual XDCR Settings out"=w180:T2)  [unwired: 10 in]
            }
          }
        }
        frame True {
          n49 = case shown="\"SUNY.rri-usa.local\", \"SUNY.rri.local\"" w222 {
            tunnel: [w251 w264 w343] -> w218
            tunnel: w221 -> [w245 w270 w364]
            tunnel: w215 -> [w225 w269 w363]
            tunnel: [w240 w268 w362] -> w216
            tunnel: w219 -> [w238 w265 w344]
            tunnel: [w236 w267 w360] -> w220
            tunnel: [w231 w266 w355] -> w214
            tunnel: ["Z8KHE" w263 "Z8KHE"] -> w217
            tunnel: [refnum<visa-resource-name> "COM7" ("JSR VISA") w261 refnum<visa-resource-name> "COM4" ("JSR VISA")] -> w212
            tunnel: [u32 1 w260 u32 1] -> w211
            frame "SUNY" {
              w235 = "G:\\"  # Data Drive
              w242 = T32 {"velocity\nmm/s"=[50.0, 2.0, 2.0], "accel\nmm/s^2"=[200.0, 4.0, 20.0]}  # Motor Parameters (Natural Units)
              w241 = i32[] [1000, 1000, 20000]  # axis steps/mm
              (unwired) refnum<visa-resource-name> "USB0::0x05FF::0x1023::3504N04910::INSTR" ("VISA resource name")
              w248 = i8 3  # # Axis
              w249 = u16 1 items=["None"=0, "Axis 1"=1, "Axis 2"=2, "Axis 3"=3, "Axis 4"=4, "Axis 5"=5, "Axis 6"=6, "Axis 7"=7, "Axis 8"=8, "Vector Space 1"=17, "Vector Space 2"=18, "Vector Space 3"=19, "Vector Space 4"=20]  # SMAC Axis
              n50 = Current VI's Path() -> (path=w229:path)
              n51 = disable-structure shown="DEPLOY==FALSE, Default" {
                disable-tunnel: w229 -> [w255 w259]
                disable-tunnel: [w253 w257] -> w228
                frame condition #0 (active) {
                  n52 = Strip Path(path=w255) -> (stripped path=w254:path)  [unwired: 1 out]
                  n53 = Build Path(base path=w254, name or relative path="StonyBrook\\DualXDCRSettingsDefault.xml") -> (appended path=w253:path)
                }
                frame condition #1 {
                  n54 = Strip Path(path=w259) -> (stripped path=w256:path)  [unwired: 1 out]
                  n55 = Build Path(base path=w256, name or relative path="data\\DualXDCRSettings.xml") -> (appended path=w257:path)
                }
              }
              n56 = Bundle By Name(cluster=w225, "Digitizer ID Cluster.ATS Ref"="ATS9350") -> (w240:T25)
              n57 = Bundle By Name(cluster=w245, "Data Drive"=w235) -> (w236:T29)
              n58 = call "MotorParam_mm_to_ct.vi"("Motor Parameters (Natural Units)"=w242, "Counts / mm"=w241) -> ("Motoar Parameters (counts)"=w247:cluster{dbl[], dbl[]})  [unwired: 9 in]
              n59 = global write "MotionGlobals.vi" "Scanning Speed Multiplier"(0.66 ("Scanning Speed Multiplier")) -> ()
              n60 = call "XDCRDefaultReader.vi"("path to XML document"=w228) -> ("Dual XDCR Settings"=w233:T2)  [unwired: 10 in]
              n61 = Bundle By Name(cluster=w238, "Motion Profile"="SMAC", "scan pair"=ScanAxis."x-(y) scan", "Reverse Z axis?"=FALSE, "SMAC Axis"=w249, "# Axis"=w248, "Steps per mm"=w241, "Motor Parameters"=w247, "Motion Bd ID"=u8 1 ("Board ID"), "overshoot cts"=500, "RT fps"=sgl 5.5) -> (w251:T22)
              n62 = Bundle By Name(cluster=w233, "Found Home"=FALSE) -> (w232:T2)
              n63 = call "SetupTimeScale.vi"("Dual XDCR Settings in"=w232) -> ("Dual XDCR Settings out"=w231:T2)  [unwired: 10 in]
            }
            frame "biomain2-n-wk.rri-usa.org", Default {
              w262 = i8 2  # Case
              n64 = case shown="1, Default" w262 {
                tunnel: w270 -> [w296 w330]
                tunnel: w269 -> [w295 w329]
                tunnel: [w294 w328] -> w268
                tunnel: [w292 w326] -> w267
                tunnel: [w287 w307] -> w266
                tunnel: w265 -> [w276 w311]
                tunnel: [w275 w310] -> w264
                tunnel: ["Z8KHE" "H0000"] -> w263
                tunnel: [refnum<visa-resource-name> "COM4" ("JSR VISA") refnum<visa-resource-name> "COM4" ("JSR VISA")] -> w261
                tunnel: [u32 1 u32 1] -> w260
                frame 1, Default {
                  w280 = i32[] [1000, 1000, 1000, 1000]  # axis steps/mm
                  w279 = T31 {"velocity mm/s"=[20.0, 20.0, 10.0, 50.0], "accel mm/s^2"=[100.0, 100.0, 50.0, 200.0]}  # Motor Parameters (Natural Units)
                  w281 = i8 4  # # Axis
                  w282 = u16 4 items=["None"=0, "Axis 1"=1, "Axis 2"=2, "Axis 3"=3, "Axis 4"=4, "Axis 5"=5, "Axis 6"=6, "Axis 7"=7, "Axis 8"=8, "Vector Space 1"=17, "Vector Space 2"=18, "Vector Space 3"=19, "Vector Space 4"=20]  # SMAC Axis
                  w291 = "F:\\"  # Data Drive
                  (unwired) refnum<visa-resource-name> "USB0::0x05FF::0x1023::3504N04910::INSTR" ("VISA resource name")
                  n65 = Current VI's Path() -> (path=w286:path)
                  n66 = disable-structure shown="DEPLOY==FALSE, Default" {
                    disable-tunnel: w286 -> [w300 w304]
                    disable-tunnel: [w297 w302] -> w285
                    frame condition #0 (active) {
                      n67 = Strip Path(path=w300) -> (stripped path=w298:path)  [unwired: 1 out]
                      n68 = Build Path(base path=w298, name or relative path="StonyBrook\\DualXDCRSettingsDebug.xml") -> (appended path=w297:path)
                    }
                    frame condition #1 {
                      n69 = Strip Path(path=w304) -> (stripped path=w301:path)  [unwired: 1 out]
                      n70 = Build Path(base path=w301, name or relative path="data\\DualXDCRSettings.xml") -> (appended path=w302:path)
                    }
                  }
                  n71 = Bundle By Name(cluster=w295, "Digitizer ID Cluster.ATS Ref"="ATS9350") -> (w294:T25)
                  n72 = Bundle By Name(cluster=w296, "Data Drive"=w291) -> (w292:T29)
                  n73 = call "MotorParam_mm_to_ct.vi"("Motor Parameters (Natural Units)"=w279, "Counts / mm"=w280) -> ("Motoar Parameters (counts)"=w278:cluster{dbl[], dbl[]})  [unwired: 9 in]
                  n74 = global write "MotionGlobals.vi" "Scanning Speed Multiplier"(0.66 ("Scanning Speed Multiplier")) -> ()
                  n75 = call "XDCRDefaultReader.vi"("path to XML document"=w285) -> ("Dual XDCR Settings"=w289:T2)  [unwired: 10 in]
                  n76 = Bundle By Name(cluster=w289, "Found Home"=FALSE) -> (w288:T2)
                  n77 = Bundle By Name(cluster=w276, "Motion Profile"="SMAC", "Reverse Z axis?"=TRUE, "SMAC Axis"=w282, "# Axis"=w281, "Steps per mm"=w280, "Motor Parameters"=w278, "scan pair"=ScanAxis."w-(y) scan") -> (w275:T22)
                  n78 = call "SetupTimeScale.vi"("Dual XDCR Settings in"=w288) -> ("Dual XDCR Settings out"=w287:T2)  [unwired: 10 in]
                }
                frame 2 {
                  w315 = i32[] [1000, 1000, 1000, 1000]  # axis steps/mm
                  w314 = T31 {"velocity mm/s"=[50.0, 20.0, 10.0, 50.0], "accel mm/s^2"=[200.0, 100.0, 50.0, 200.0]}  # Motor Parameters (Natural Units)
                  w316 = i8 4  # # Axis
                  w317 = u16 4 items=["None"=0, "Axis 1"=1, "Axis 2"=2, "Axis 3"=3, "Axis 4"=4, "Axis 5"=5, "Axis 6"=6, "Axis 7"=7, "Axis 8"=8, "Vector Space 1"=17, "Vector Space 2"=18, "Vector Space 3"=19, "Vector Space 4"=20]  # SMAC Axis
                  w325 = "F:\\"  # Data Drive
                  (unwired) refnum<visa-resource-name> "USB0::0x05FF::0x1023::3504N04910::INSTR" ("VISA resource name")
                  n79 = Current VI's Path() -> (path=w321:path)
                  n80 = disable-structure shown="DEPLOY==FALSE, Default" {
                    disable-tunnel: w321 -> [w334 w338]
                    disable-tunnel: [w331 w336] -> w320
                    frame condition #0 (active) {
                      n81 = Strip Path(path=w334) -> (stripped path=w332:path)  [unwired: 1 out]
                      n82 = Build Path(base path=w332, name or relative path="StonyBrook\\DualXDCRSettingsDebug.xml") -> (appended path=w331:path)
                    }
                    frame condition #1 {
                      n83 = Strip Path(path=w338) -> (stripped path=w335:path)  [unwired: 1 out]
                      n84 = Build Path(base path=w335, name or relative path="data\\DualXDCRSettings.xml") -> (appended path=w336:path)
                    }
                  }
                  n85 = Bundle By Name(cluster=w329, "Digitizer ID Cluster.ATS Ref"="ATS9350") -> (w328:T25)
                  n86 = Bundle By Name(cluster=w330, "Data Drive"=w325) -> (w326:T29)
                  n87 = call "MotorParam_mm_to_ct.vi"("Motor Parameters (Natural Units)"=w314, "Counts / mm"=w315) -> ("Motoar Parameters (counts)"=w313:cluster{dbl[], dbl[]})  [unwired: 9 in]
                  n88 = global write "MotionGlobals.vi" "Scanning Speed Multiplier"(0.66 ("Scanning Speed Multiplier")) -> ()
                  n89 = call "XDCRDefaultReader.vi"("path to XML document"=w320) -> ("Dual XDCR Settings"=w323:T2)  [unwired: 10 in]
                  n90 = Bundle By Name(cluster=w323, "Found Home"=FALSE) -> (w322:T2)
                  n91 = Bundle By Name(cluster=w311, "Motion Profile"="StonyTest", "Reverse Z axis?"=TRUE, "SMAC Axis"=w317, "# Axis"=w316, "Steps per mm"=w315, "Motor Parameters"=w313, "scan pair"=ScanAxis."x-(y) scan") -> (w310:T22)
                  n92 = call "SetupTimeScale.vi"("Dual XDCR Settings in"=w322) -> ("Dual XDCR Settings out"=w307:T2)  [unwired: 10 in]
                }
              }
            }
            frame "SUNY.rri-usa.local", "SUNY.rri.local" {
              w348 = i32[] [1000, 1000, 1000]  # axis steps/mm
              w347 = T31 {"velocity mm/s"=[50.0, 20.0, 20.0], "accel mm/s^2"=[200.0, 100.0, 100.0]}  # Motor Parameters (Natural Units)
              w349 = i8 3  # # Axis
              w350 = u16 1 items=["None"=0, "Axis 1"=1, "Axis 2"=2, "Axis 3"=3, "Axis 4"=4, "Axis 5"=5, "Axis 6"=6, "Axis 7"=7, "Axis 8"=8, "Vector Space 1"=17, "Vector Space 2"=18, "Vector Space 3"=19, "Vector Space 4"=20]  # SMAC Axis
              w359 = "G:\\"  # Data Drive
              (unwired) refnum<visa-resource-name> "USB0::0x05FF::0x1023::3504N04910::INSTR" ("VISA resource name")
              n93 = Current VI's Path() -> (path=w354:path)
              n94 = disable-structure shown="DEPLOY==FALSE, Default" {
                disable-tunnel: w354 -> [w368 w372]
                disable-tunnel: [w365 w370] -> w353
                frame condition #0 (active) {
                  n95 = Strip Path(path=w368) -> (stripped path=w366:path)  [unwired: 1 out]
                  n96 = Build Path(base path=w366, name or relative path="StonyBrook\\DualXDCRSettingsDebug.xml") -> (appended path=w365:path)
                }
                frame condition #1 {
                  n97 = Strip Path(path=w372) -> (stripped path=w369:path)  [unwired: 1 out]
                  n98 = Build Path(base path=w369, name or relative path="data\\DualXDCRSettings.xml") -> (appended path=w370:path)
                }
              }
              n99 = Bundle By Name(cluster=w363, "Digitizer ID Cluster.ATS Ref"="ATS9350") -> (w362:T25)
              n100 = Bundle By Name(cluster=w364, "Data Drive"=w359) -> (w360:T29)
              n101 = call "MotorParam_mm_to_ct.vi"("Motor Parameters (Natural Units)"=w347, "Counts / mm"=w348) -> ("Motoar Parameters (counts)"=w346:cluster{dbl[], dbl[]})  [unwired: 9 in]
              n102 = global write "MotionGlobals.vi" "Scanning Speed Multiplier"(0.66 ("Scanning Speed Multiplier")) -> ()
              n103 = call "XDCRDefaultReader.vi"("path to XML document"=w353) -> ("Dual XDCR Settings"=w357:T2)  [unwired: 10 in]
              n104 = Bundle By Name(cluster=w357, "Found Home"=FALSE) -> (w356:T2)
              n105 = Bundle By Name(cluster=w344, "Motion Profile"="SMAC", "Reverse Z axis?"=FALSE, "SMAC Axis"=w350, "# Axis"=w349, "Steps per mm"=w348, "Motor Parameters"=w346, "scan pair"=ScanAxis."x-(y) scan") -> (w343:T22)
              n106 = call "SetupTimeScale.vi"("Dual XDCR Settings in"=w356) -> ("Dual XDCR Settings out"=w355:T2)  [unwired: 10 in]
            }
          }
        }
      }
    }
    frame "WCM Rotation" {
      (unwired) "PCI::SER19507" ("ResourceName")
      n107 = case shown="\"PC305435.a.wcmc-ad.net\"" w374 {
        tunnel: [w387 w395] -> w379
        tunnel: w378 -> [w386 w394]
        frame Default {
          w382 = i32[] [1000, 4000, 2000, 1000]  # axis steps/mm
          w383 = T31 {"velocity mm/s"=[10.0, 4.0, 2.0, 50.0], "accel mm/s^2"=[50.0, 50.0, 20.0, 200.0]}  # Motor Parameters (Natural Units)
          (unwired) refnum<visa-resource-name> "USB0::0x05FF::0x1023::3504N04910::INSTR" ("VISA resource name")
          w384 = i8 4  # # Axis
          w385 = u16 4 items=["None"=0, "Axis 1"=1, "Axis 2"=2, "Axis 3"=3, "Axis 4"=4, "Axis 5"=5, "Axis 6"=6, "Axis 7"=7, "Axis 8"=8, "Vector Space 1"=17, "Vector Space 2"=18, "Vector Space 3"=19, "Vector Space 4"=20]  # SMAC Axis
          n108 = call "MotorParam_mm_to_ct.vi"("Motor Parameters (Natural Units)"=w383, "Counts / mm"=w382) -> ("Motoar Parameters (counts)"=w381:cluster{dbl[], dbl[]})  [unwired: 9 in]
          n109 = Bundle By Name(cluster=w386, "SMAC Axis"=w385, "# Axis"=w384, "Steps per mm"=w382, "Motor Parameters"=w381, "Motion Profile"="SMAC Rotation") -> (w387:T22)
        }
        frame "PC305435.a.wcmc-ad.net" {
          w391 = i32[] [4000, 4000, 2000, 1000]  # axis steps/mm
          w392 = T31 {"velocity mm/s"=[10.0, 4.0, 2.0, 50.0], "accel mm/s^2"=[50.0, 50.0, 20.0, 200.0]}  # Motor Parameters (Natural Units)
          (unwired) refnum<visa-resource-name> "USB0::0x05FF::0x1023::3504N04910::INSTR" ("VISA resource name")
          w393 = i8 1  # # Axis
          (unwired) u16 5 items=["None"=0, "Axis 1"=1, "Axis 2"=2, "Axis 3"=3, "Axis 4"=4, "Axis 5"=5, "Axis 6"=6, "Axis 7"=7, "Axis 8"=8, "Vector Space 1"=17, "Vector Space 2"=18, "Vector Space 3"=19, "Vector Space 4"=20]  # SMAC Axis
          n110 = call "MotorParam_mm_to_ct.vi"("Motor Parameters (Natural Units)"=w392, "Counts / mm"=w391) -> ("Motoar Parameters (counts)"=w390:cluster{dbl[], dbl[]})  [unwired: 9 in]
          n111 = Bundle By Name(cluster=w394, "# Axis"=w393, "Steps per mm"=w391, "Motor Parameters"=w390, "Motion Profile"="Single Axis Rotation", "Galil Address"="192.168.42.2") -> (w395:T22)
        }
      }
    }
    frame "WCM Microscopy" {
      w405 = sgl 2.0 ("Distance between\nscan lines (um)")
      w399 = TRUE ("One Way Scan")
      w409 = "D:\\"  # Data Drive
      w414 = T31 {"velocity mm/s"=[30.0, 30.0, 2.0, 75.0], "accel mm/s^2"=[125.0, 125.0, 10.0, 250.0]}  # Motor Parameters (Natural Units)
      w413 = i32[] [1000, 1000, 50802, 1000]  # axis steps/mm
      w416 = i8 3  # # Axis
      w415 = u16 0 items=["None"=0, "Axis 1"=1, "Axis 2"=2, "Axis 3"=3, "Axis 4"=4, "Axis 5"=5, "Axis 6"=6, "Axis 7"=7, "Axis 8"=8, "Vector Space 1"=17, "Vector Space 2"=18, "Vector Space 3"=19, "Vector Space 4"=20]  # SMAC Axis
      (unwired) "PCI::SER19507" ("ResourceName")
      n112 = Bundle By Name(cluster=w411, "Data Drive"=w409, "Tabor Address"="Tabor2182") -> (w410:T29)
      n113 = Bundle By Name(cluster=w408, "Digitizer ID Cluster.LeCroy VISA"="Microscopy Scope", "lines per plane"=101, "rf points per line"=200) -> (w401:T25)
      n114 = call "MotorParam_mm_to_ct.vi"("Motor Parameters (Natural Units)"=w414, "Counts / mm"=w413) -> ("Motoar Parameters (counts)"=w412:cluster{dbl[], dbl[]})  [unwired: 9 in]
      n115 = Bundle By Name(cluster=w417, "Reverse Z axis?"=FALSE, "SMAC Axis"=w415, "# Axis"=w416, "Steps per mm"=w413, "Motor Parameters"=w412, "Motion Profile"="SAM Smooth", "One Way Scan"=w399, "Reverse One Way Scan"=w399, "Distance between\nscan lines (um)"=w405, "Distance between\nscan planes (um)"=w405, "number of scan planes"=1, "scan pair"=ScanAxis."x-(y) scan") -> (w418:T22)
    }
    frame "WCM SAM SMAC" {
      w429 = sgl 2.0 ("Distance between\nscan lines (um)")
      w423 = TRUE ("One Way Scan")
      w433 = "E:\\"  # Data Drive
      w438 = T31 {"velocity mm/s"=[50.0, 50.0, 2.0, 75.0], "accel mm/s^2"=[200.0, 200.0, 10.0, 250.0]}  # Motor Parameters (Natural Units)
      w437 = i32[] [10000, 10000, 50802, 1000]  # axis steps/mm
      w440 = i8 3  # # Axis
      w439 = u16 0 items=["None"=0, "Axis 1"=1, "Axis 2"=2, "Axis 3"=3, "Axis 4"=4, "Axis 5"=5, "Axis 6"=6, "Axis 7"=7, "Axis 8"=8, "Vector Space 1"=17, "Vector Space 2"=18, "Vector Space 3"=19, "Vector Space 4"=20]  # SMAC Axis
      (unwired) "PCI::SER19507" ("ResourceName")
      n116 = Bundle By Name(cluster=w435, "Data Drive"=w433, "Tabor Address"="Tabor2182") -> (w434:T29)
      n117 = Bundle By Name(cluster=w432, "Digitizer ID Cluster.LeCroy VISA"="Microscopy Scope 2", "lines per plane"=101, "rf points per line"=200) -> (w425:T25)
      n118 = call "MotorParam_mm_to_ct.vi"("Motor Parameters (Natural Units)"=w438, "Counts / mm"=w437) -> ("Motoar Parameters (counts)"=w436:cluster{dbl[], dbl[]})  [unwired: 9 in]
      n119 = Bundle By Name(cluster=w441, "Reverse Z axis?"=FALSE, "SMAC Axis"=w439, "# Axis"=w440, "Steps per mm"=w437, "Motor Parameters"=w436, "Motion Profile"="XY_Stage", "One Way Scan"=w423, "Reverse One Way Scan"=w423, "Distance between\nscan lines (um)"=w429, "Distance between\nscan planes (um)"=w429, "number of scan planes"=1, "scan pair"=ScanAxis."x-(y) scan") -> (w442:T22)
    }
    frame "SERI SAM 2023" {
      w454 = sgl 2.0 ("Distance between\nscan lines (um)")
      w448 = TRUE ("One Way Scan")
      w457 = "E:\\"  # Data Drive
      w462 = T31 {"velocity mm/s"=[50.0, 50.0, 2.0, 75.0], "accel mm/s^2"=[200.0, 200.0, 10.0, 250.0]}  # Motor Parameters (Natural Units)
      w461 = i32[] [10000, 10000, 50802, 1000]  # axis steps/mm
      w464 = i8 3  # # Axis
      w463 = u16 0 items=["None"=0, "Axis 1"=1, "Axis 2"=2, "Axis 3"=3, "Axis 4"=4, "Axis 5"=5, "Axis 6"=6, "Axis 7"=7, "Axis 8"=8, "Vector Space 1"=17, "Vector Space 2"=18, "Vector Space 3"=19, "Vector Space 4"=20]  # SMAC Axis
      (unwired) "PCI::SER19507" ("ResourceName")
      n120 = Bundle By Name(cluster=w459, "Data Drive"=w457, "Tabor Address"="Tabor2182") -> (w458:T29)
      n121 = Bundle By Name(cluster=w456, "lines per plane"=101, "rf points per line"=200) -> (w450:T25)
      n122 = call "MotorParam_mm_to_ct.vi"("Motor Parameters (Natural Units)"=w462, "Counts / mm"=w461) -> ("Motoar Parameters (counts)"=w460:cluster{dbl[], dbl[]})  [unwired: 9 in]
      n123 = Bundle By Name(cluster=w465, "Reverse Z axis?"=FALSE, "SMAC Axis"=w463, "# Axis"=w464, "Steps per mm"=w461, "Motor Parameters"=w460, "Motion Profile"="SMAC", "One Way Scan"=w448, "Reverse One Way Scan"=w448, "Distance between\nscan lines (um)"=w454, "Distance between\nscan planes (um)"=w454, "number of scan planes"=1, "scan pair"=ScanAxis."x-(y) scan", "Galil Address"="192.168.1.100") -> (w466:T22)
    }
    frame "WCM Main 2Axis" {
      w474 = T31 {"velocity mm/s"=[10.0, 10.0, 10.0, 50.0], "accel mm/s^2"=[50.0, 50.0, 50.0, 200.0]}  # Motor Parameters (Natural Units)
      w475 = i32[] [2000, 1000, 1000, 1000]
      (unwired) refnum<visa-resource-name> "USB0::0x05FF::0x1023::3504N04910::INSTR" ("VISA resource name")
      w478 = i8 4  # # Axis
      w479 = u16 4 items=["None"=0, "Axis 1"=1, "Axis 2"=2, "Axis 3"=3, "Axis 4"=4, "Axis 5"=5, "Axis 6"=6, "Axis 7"=7, "Axis 8"=8, "Vector Space 1"=17, "Vector Space 2"=18, "Vector Space 3"=19, "Vector Space 4"=20]  # SMAC Axis
      (unwired) "PCI::SER19507" ("ResourceName")
      n124 = call "MotorParam_mm_to_ct.vi"("Motor Parameters (Natural Units)"=w474, "Counts / mm"=w475) -> ("Motoar Parameters (counts)"=w477:cluster{dbl[], dbl[]})  [unwired: 9 in]
      n125 = Bundle By Name(cluster=w470, "SMAC Axis"=w479, "# Axis"=w478, "Steps per mm"=w475, "Motor Parameters"=w477, "Motion Profile"="SMAC 2Axi") -> (w476:T22)
    }
    frame "WCM Optics Lab" {
      w488 = T31 {"velocity mm/s"=[0.5, 10.0, 10.0, 50.0], "accel mm/s^2"=[5.0, 50.0, 50.0, 200.0]}  # Motor Parameters (Natural Units)
      w487 = i32[] [2000, 1000, 1000, 1000]
      (unwired) refnum<visa-resource-name> "USB0::0x05FF::0x1023::3504N04910::INSTR" ("VISA resource name")
      w491 = i8 4  # # Axis
      w492 = u16 4 items=["None"=0, "Axis 1"=1, "Axis 2"=2, "Axis 3"=3, "Axis 4"=4, "Axis 5"=5, "Axis 6"=6, "Axis 7"=7, "Axis 8"=8, "Vector Space 1"=17, "Vector Space 2"=18, "Vector Space 3"=19, "Vector Space 4"=20]  # SMAC Axis
      (unwired) "PCI::SER19507" ("ResourceName")
      n126 = call "MotorParam_mm_to_ct.vi"("Motor Parameters (Natural Units)"=w488, "Counts / mm"=w487) -> ("Motoar Parameters (counts)"=w486:cluster{dbl[], dbl[]})  [unwired: 9 in]
      n127 = Bundle By Name(cluster=w489, "SMAC Axis"=w492, "# Axis"=w491, "Steps per mm"=w487, "Motor Parameters"=w486, "Motion Profile"="SMAC", "Galil Address"="192.168.42.3" ("For Galil")) -> (w490:T22)
    }
    frame "Hawaii" {
      n128 = case shown="True" w494 {
        tunnel: w503 -> [w535 w553]
        tunnel: w502 -> [w531 w552]
        tunnel: [w530 w551] -> w501
        tunnel: w500 -> [w527 w550]
        tunnel: [w510 w549] -> w499
        tunnel: [w509 w548] -> w498
        tunnel: [w508 w547] -> w497
        tunnel: ["H0000" w546] -> w496
        tunnel: [refnum<visa-resource-name> "GPIB0::1::INSTR" ("VISA resource name") w545] -> w495
        tunnel: w493 -> [_ w544]
        frame False {
          (unwired) "Hawaii\\DualXDCRSettingsDebug.xml" ("name or relative path")
          w507 = u16 0 items=["None"=0, "Axis 1"=1, "Axis 2"=2, "Axis 3"=3, "Axis 4"=4, "Axis 5"=5, "Axis 6"=6, "Axis 7"=7, "Axis 8"=8, "Vector Space 1"=17, "Vector Space 2"=18, "Vector Space 3"=19, "Vector Space 4"=20]  # SMAC Axis
          w522 = sgl 50.0 ("Distance between\nscan lines (um)")
          w523 = T31 {"velocity mm/s"=[20.0, 20.0, 20.0], "accel mm/s^2"=[200.0, 200.0, 200.0]}  # Motor Parameters (Natural Units)
          w529 = "E:\\"  # Data Drive
          w533 = i32[] [2000, 2000, 2000, 2000]  # Axis Counts/mm
          w534 = i8 3  # # Axis
          # "Dr. Machi's System Aerotech"
          n129 = Current VI's Path() -> (path=w512:path)
          n130 = disable-structure shown="DEPLOY==FALSE, Default" {
            disable-tunnel: w512 -> [w539 w543]
            disable-tunnel: [w537 w541] -> w511
            frame condition #0 (active) {
              n131 = Strip Path(path=w539) -> (stripped path=w538:path)  [unwired: 1 out]
              n132 = Build Path(base path=w538, name or relative path="Hawaii\\DualXDCRSettingsDefault.xml") -> (appended path=w537:path)
            }
            frame condition #1 {
              n133 = Strip Path(path=w543) -> (stripped path=w540:path)  [unwired: 1 out]
              n134 = Build Path(base path=w540, name or relative path="data\\DualXDCRSettings.xml") -> (appended path=w541:path)
            }
          }
          n135 = Bundle By Name(cluster=w531, "Data Drive"=w529, "Tabor Address"="ASRL3::INSTR" ("resource name")) -> (w530:T29)
          n136 = call "MotorParam_mm_to_ct.vi"("Motor Parameters (Natural Units)"=w523, "Counts / mm"=w533) -> ("Motoar Parameters (counts)"=w532:cluster{dbl[], dbl[]})  [unwired: 9 in]
          n137 = Bundle By Name(cluster=w527, "Digitizer ID Cluster.LeCroy VISA"=refnum<visa-resource-name> "USB0::0x05FF::0x1023::3504N04910::INSTR" ("VISA resource name"), "Voltage Scale"=0.5, "lines per plane"=101, "rf points per line"=512, "Digitizer delay (us)"=2.0, "Samp Rate (Hz)"=250000000.0) -> (w510:T25)
          n138 = Bundle By Name(cluster=w535, "# Axis"=w534, "Steps per mm"=w533, "Motor Parameters"=w532, "Motion Profile"="AeroTechTest", "Distance between\nscan lines (um)"=w522, "Distance between\nscan planes (um)"=w522, "number of scan planes"=1, "RT fps"=sgl 6.0, "SMAC Axis"=w507, "scan pair"=ScanAxis."x-(y) scan") -> (w509:T22)
          n139 = call "XDCRDefaultReader.vi"("path to XML document"=w511) -> ("Dual XDCR Settings"=w514:T2)  [unwired: 10 in]
          n140 = Bundle By Name(cluster=w514, "Found Home"=FALSE) -> (w513:T2)
          n141 = call "SetupTimeScale.vi"("Dual XDCR Settings in"=w513) -> ("Dual XDCR Settings out"=w508:T2)  [unwired: 10 in]
        }
        frame True {
          n142 = case shown="\"biomain2-n-wk.rri-usa.org\"" w544 {
            tunnel: w553 -> [w586 w630]
            tunnel: w552 -> [w582 w626]
            tunnel: [w581 w625] -> w551
            tunnel: w550 -> [w578 w622]
            tunnel: [w561 w605] -> w549
            tunnel: [w560 w604] -> w548
            tunnel: [w559 w603] -> w547
            tunnel: ["H0000" "H0000"] -> w546
            tunnel: [refnum<visa-resource-name> "GPIB0::1::INSTR" ("VISA resource name") refnum<visa-resource-name> "GPIB0::1::INSTR" ("VISA resource name")] -> w545
            frame "Hawaii-wk.rri.local", Default {
              (unwired) "Hawaii\\DualXDCRSettingsDebug.xml" ("name or relative path")
              w558 = u16 0 items=["None"=0, "Axis 1"=1, "Axis 2"=2, "Axis 3"=3, "Axis 4"=4, "Axis 5"=5, "Axis 6"=6, "Axis 7"=7, "Axis 8"=8, "Vector Space 1"=17, "Vector Space 2"=18, "Vector Space 3"=19, "Vector Space 4"=20]  # SMAC Axis
              w573 = sgl 50.0 ("Distance between\nscan lines (um)")
              w574 = T31 {"velocity mm/s"=[20.0, 20.0, 20.0], "accel mm/s^2"=[200.0, 200.0, 200.0]}  # Motor Parameters (Natural Units)
              w580 = "E:\\"  # Data Drive
              w584 = i32[] [2000, 2000, 2000, 2000]  # Axis Counts/mm
              w585 = i8 3  # # Axis
              # "Dr. Machi's System Aerotech"
              n143 = Current VI's Path() -> (path=w563:path)
              n144 = disable-structure shown="DEPLOY==FALSE, Default" {
                disable-tunnel: w563 -> [w593 w597]
                disable-tunnel: [w590 w595] -> w562
                frame condition #0 (active) {
                  n145 = Strip Path(path=w593) -> (stripped path=w591:path)  [unwired: 1 out]
                  n146 = Build Path(base path=w591, name or relative path="Hawaii\\DualXDCRSettingsDebug.xml") -> (appended path=w590:path)
                }
                frame condition #1 {
                  n147 = Strip Path(path=w597) -> (stripped path=w594:path)  [unwired: 1 out]
                  n148 = Build Path(base path=w594, name or relative path="data\\DualXDCRSettings.xml") -> (appended path=w595:path)
                }
              }
              n149 = Bundle By Name(cluster=w582, "Data Drive"=w580, "Tabor Address"="ASRL3::INSTR" ("resource name")) -> (w581:T29)
              n150 = call "MotorParam_mm_to_ct.vi"("Motor Parameters (Natural Units)"=w574, "Counts / mm"=w584) -> ("Motoar Parameters (counts)"=w583:cluster{dbl[], dbl[]})  [unwired: 9 in]
              n151 = Bundle By Name(cluster=w578, "Digitizer ID Cluster.LeCroy VISA"=refnum<visa-resource-name> "USB0::0x05FF::0x1023::3504N04910::INSTR" ("VISA resource name"), "Voltage Scale"=0.5, "lines per plane"=101, "rf points per line"=512, "Digitizer delay (us)"=2.0, "Samp Rate (Hz)"=250000000.0) -> (w561:T25)
              n152 = Bundle By Name(cluster=w586, "# Axis"=w585, "Steps per mm"=w584, "Motor Parameters"=w583, "Motion Profile"="AeroTechTest", "Distance between\nscan lines (um)"=w573, "Distance between\nscan planes (um)"=w573, "number of scan planes"=1, "RT fps"=sgl 6.0, "SMAC Axis"=w558, "scan pair"=ScanAxis."x-(y) scan") -> (w560:T22)
              n153 = call "XDCRDefaultReader.vi"("path to XML document"=w562) -> ("Dual XDCR Settings"=w565:T2)  [unwired: 10 in]
              n154 = Bundle By Name(cluster=w565, "Found Home"=FALSE) -> (w564:T2)
              n155 = case shown="True" TRUE {
                tunnel: w564 -> [w587 w589]
                tunnel: [w587 w588] -> w559
                frame False {
                }
                frame True {
                  n156 = call "SetupTimeScale.vi"("Dual XDCR Settings in"=w589) -> ("Dual XDCR Settings out"=w588:T2)  [unwired: 10 in]
                }
              }
            }
            frame "biomain2-n-wk.rri-usa.org" {
              (unwired) "Hawaii\\DualXDCRSettingsDebug.xml" ("name or relative path")
              w602 = u16 0 items=["None"=0, "Axis 1"=1, "Axis 2"=2, "Axis 3"=3, "Axis 4"=4, "Axis 5"=5, "Axis 6"=6, "Axis 7"=7, "Axis 8"=8, "Vector Space 1"=17, "Vector Space 2"=18, "Vector Space 3"=19, "Vector Space 4"=20]  # SMAC Axis
              w617 = sgl 50.0 ("Distance between\nscan lines (um)")
              w618 = T31 {"velocity mm/s"=[20.0, 20.0, 20.0], "accel mm/s^2"=[200.0, 200.0, 200.0]}  # Motor Parameters (Natural Units)
              w624 = "F:\\"  # Data Drive
              w628 = i32[] [1000, 1000, 1000, 1000]  # Axis Counts/mm
              w629 = i8 3  # # Axis
              # "Dr. Machi's System Aerotech"
              n157 = Current VI's Path() -> (path=w607:path)
              n158 = disable-structure shown="DEPLOY==FALSE, Default" {
                disable-tunnel: w607 -> [w637 w641]
                disable-tunnel: [w634 w639] -> w606
                frame condition #0 (active) {
                  n159 = Strip Path(path=w637) -> (stripped path=w635:path)  [unwired: 1 out]
                  n160 = Build Path(base path=w635, name or relative path="Hawaii\\DualXDCRSettingsDefault.xml") -> (appended path=w634:path)
                }
                frame condition #1 {
                  n161 = Strip Path(path=w641) -> (stripped path=w638:path)  [unwired: 1 out]
                  n162 = Build Path(base path=w638, name or relative path="data\\DualXDCRSettings.xml") -> (appended path=w639:path)
                }
              }
              n163 = Bundle By Name(cluster=w626, "Data Drive"=w624, "Tabor Address"="ASRL3::INSTR" ("resource name")) -> (w625:T29)
              n164 = call "MotorParam_mm_to_ct.vi"("Motor Parameters (Natural Units)"=w618, "Counts / mm"=w628) -> ("Motoar Parameters (counts)"=w627:cluster{dbl[], dbl[]})  [unwired: 9 in]
              n165 = Bundle By Name(cluster=w622, "Digitizer ID Cluster.LeCroy VISA"=refnum<visa-resource-name> "USB0::0x05FF::0x1023::3504N04910::INSTR" ("VISA resource name"), "Voltage Scale"=0.5, "lines per plane"=101, "rf points per line"=512, "Digitizer delay (us)"=2.0, "Samp Rate (Hz)"=250000000.0) -> (w605:T25)
              n166 = Bundle By Name(cluster=w630, "# Axis"=w629, "Steps per mm"=w628, "Motor Parameters"=w627, "Motion Profile"="SMAC", "Distance between\nscan lines (um)"=w617, "Distance between\nscan planes (um)"=w617, "number of scan planes"=1, "RT fps"=sgl 6.0, "SMAC Axis"=w602, "scan pair"=ScanAxis."x-(y) scan") -> (w604:T22)
              n167 = call "XDCRDefaultReader.vi"("path to XML document"=w606) -> ("Dual XDCR Settings"=w609:T2)  [unwired: 10 in]
              n168 = Bundle By Name(cluster=w609, "Found Home"=FALSE) -> (w608:T2)
              n169 = case shown="True" TRUE {
                tunnel: w608 -> [w631 w633]
                tunnel: [w631 w632] -> w603
                frame False {
                }
                frame True {
                  n170 = call "SetupTimeScale.vi"("Dual XDCR Settings in"=w633) -> ("Dual XDCR Settings out"=w632:T2)  [unwired: 10 in]
                }
              }
            }
          }
        }
      }
    }
    frame "Columbia  NI System" {
      w647 = "D:\\"  # Data Drive
      w651 = T31 {"velocity mm/s"=[10.0, 10.0, 10.0, 50.0], "accel mm/s^2"=[50.0, 50.0, 50.0, 200.0]}  # Motor Parameters (Natural Units)
      w653 = i32[] [1000, 1000, 1000, 1000]  # axis steps/mm
      w656 = i8 3  # # Axis
      (unwired) "PCI::INSTR1" ("Resource Name (PCI::INSTR0)")
      n171 = Bundle By Name(cluster=w646, "Digitizer ID Cluster.ATS Ref"="ATS9440" ("BoardToVerify")) -> (w645:T25)
      n172 = Bundle By Name(cluster=w650, "Data Drive"=w647, "Tabor Address"="ASRL3::INSTR" ("resource name")) -> (w649:T29)
      n173 = call "MotorParam_mm_to_ct.vi"("Motor Parameters (Natural Units)"=w651, "Counts / mm"=w653) -> ("Motoar Parameters (counts)"=w652:cluster{dbl[], dbl[]})  [unwired: 9 in]
      n174 = Bundle By Name(cluster=w654, "# Axis"=w656, "Steps per mm"=w653, "Motor Parameters"=w652, "Motion Profile"="SMAC") -> (w655:T22)
    }
    frame "CUMC RT" {
      w667 = "F:\\"  # Data Drive
      w671 = T31 {"velocity mm/s"=[10.0, 10.0, 10.0, 50.0], "accel mm/s^2"=[50.0, 50.0, 50.0, 200.0]}  # Motor Parameters (Natural Units)
      w673 = i32[] [1000, 1000, 1000, 1000]  # axis steps/mm
      w676 = i8 3  # # Axis
      (unwired) "PCI::INSTR1" ("Resource Name (PCI::INSTR0)")
      n175 = Bundle By Name(cluster=w666, "Digitizer ID Cluster.ATS Ref"="ATS9440" ("BoardToVerify")) -> (w665:T25)
      n176 = Bundle By Name(cluster=w670, "Data Drive"=w667, "Tabor Address"="ASRL3::INSTR" ("resource name")) -> (w669:T29)
      n177 = call "MotorParam_mm_to_ct.vi"("Motor Parameters (Natural Units)"=w671, "Counts / mm"=w673) -> ("Motoar Parameters (counts)"=w672:cluster{dbl[], dbl[]})  [unwired: 9 in]
      n178 = Bundle By Name(cluster=w674, "No Motion?"=TRUE, "# Axis"=w676, "Steps per mm"=w673, "Motor Parameters"=w672, "Motion Profile"="SMAC", "number of scan planes"=1, "Distance between\nscan lines (um)"=sgl 50.0 ("Distance between\nscan lines (um)"), "Distance between\nscan planes (um)"=sgl 50.0 ("Distance between\nscan planes (um)")) -> (w675:T22)
    }
    frame "NYU" {
      w696 = T31 {"velocity mm/s"=[50.0, 10.0], "accel mm/s^2"=[200.0, 50.0]}  # Motor Parameters (Natural Units)
      w697 = i32[] [1000, 1000]  # axis counts/mm
      w701 = i8 2  # # Axis
      w702 = u16 1 items=["None"=0, "Axis 1"=1, "Axis 2"=2, "Axis 3"=3, "Axis 4"=4, "Axis 5"=5, "Axis 6"=6, "Axis 7"=7, "Axis 8"=8, "Vector Space 1"=17, "Vector Space 2"=18, "Vector Space 3"=19, "Vector Space 4"=20]  # SMAC Axis
      n179 = case shown="False" FALSE {
        tunnel: [TRUE ("T button?") w704] -> w682
        frame False {
        }
        frame True {
          n180 = Two Button Dialog(message="Where would you like to save the data?", 1:"OARIST-PC" ("F button name (\"Cancel\")"), 2:"Locally" ("T button name (\"OK\")")) -> (T button?=w704:bool)
        }
      }
      n181 = Select(t="C:\\" ("Data Drive"), s=w682, f="\\\\OARIST-PC\\Annular Array\\") -> (s? t:f=w684:string)
      n182 = Bundle By Name(cluster=w693, "Tabor Address"="ASRL3::INSTR" ("resource name"), "Data Drive"=w684) -> (w694:T29)
      n183 = call "MotorParam_mm_to_ct.vi"("Motor Parameters (Natural Units)"=w696, "Counts / mm"=w697) -> ("Motoar Parameters (counts)"=w698:cluster{dbl[], dbl[]})  [unwired: 9 in]
      n184 = Bundle By Name(cluster=w699, "SMAC Axis"=w702, "# Axis"=w701, "Steps per mm"=w697, "Motor Parameters"=w698, "Motion Profile"="SMAC 2Axis", "Galil Address"="192.168.42.3" ("For Galil")) -> (w700:T22)
      n185 = Bundle By Name(cluster=w692, "Digitizer delay (us)"=7.0, "rf points per line"=3000, "lines per plane"=161, "Samp Rate (Hz)"=250000000.0) -> (w689:T25)
    }
    frame "UHI Allen" {
      w713 = "D:\\"  # Data Drive
      w717 = i32[] [1000, 10000, 1000]  # ESP Ct/mm
      w718 = i8 3  # # Axis
      # "John's HI ESP300 system."
      n186 = VISA Open(access mode=u32 0, VISA resource name=refnum<visa-resource-name> "GPIB0::2::INSTR") -> (VISA resource name=w722:refnum<visa-resource-name>, error out=w723:errorcluster)  [unwired: 3 in]
      n187 = Bundle By Name(cluster=w711, "Data Drive"=w713, "Tabor Address"="ASRL3::INSTR" ("resource name")) -> (w710:T29)
      n188 = VISA Clear(VISA resource name=w722, error in (no error)=w723) -> (VISA resource name out=w714:refnum<visa-resource-name>)  [unwired: 1 out]
      n189 = Bundle By Name(cluster=w715, "# Axis"=w718, "Steps per mm"=w717, "ESP VISA"=w714) -> (w716:T22)
    }
    frame "Chiba" {
      w733 = "D:\\"  # Data Drive
      w736 = T31 {"velocity mm/s"=[10.0, 10.0, 10.0], "accel mm/s^2"=[50.0, 50.0, 50.0]}  # Motor Parameters (Natural Units)
      w737 = i32[] [5000, 5000, 10000]  # axis steps/mm
      (unwired) refnum<visa-resource-name> "VICP::LCRY0310M26683"  # Chiba V44MX
      (unwired) refnum<visa-resource-name> "VICP::LCRY0604P15336"  # Chiba 6030
      (unwired) refnum<visa-resource-name> "VICP::LCRY0602P10739" ("VISA resource name")
      w739 = i8 3  # # Axis
      w740 = u16 0 items=["None"=0, "Axis 1"=1, "Axis 2"=2, "Axis 3"=3, "Axis 4"=4, "Axis 5"=5, "Axis 6"=6, "Axis 7"=7, "Axis 8"=8, "Vector Space 1"=17, "Vector Space 2"=18, "Vector Space 3"=19, "Vector Space 4"=20]  # SMAC Axis
      (unwired) "PCI::SER19507" ("ResourceName")
      n190 = Bundle By Name(cluster=w729, "Digitizer ID Cluster.LeCroy VISA"="LeCroy IP Address") -> (w727:T25)
      n191 = Bundle By Name(cluster=w731, "Data Drive"=w733, "Tabor Address"="ASRL3::INSTR" ("resource name")) -> (w732:T29)
      n192 = call "MotorParam_mm_to_ct.vi"("Motor Parameters (Natural Units)"=w736, "Counts / mm"=w737) -> ("Motoar Parameters (counts)"=w735:cluster{dbl[], dbl[]})  [unwired: 9 in]
      n193 = Bundle By Name(cluster=w730, "SMAC Axis"=w740, "# Axis"=w739, "Steps per mm"=w737, "Motor Parameters"=w735, "Motion Profile"="SMAC", "Galil Address"="192.168.42.2" ("For Galil")) -> (w738:T22)
    }
  }
  "Motion Settings" <- w23
  "Bypass 2nd dig init" <- w29
  "Digitizer Settings" <- w22
  "Hardware Addresses" <- w27
  "Dual XDCR Settings" <- w8
  "Switch T/R" <- w4
  n194 = global write "PulserGlobals.vi" "UTEX VISA"(w2) -> ()
  n195 = Unbundle By Name(w27) -> ("Data Drive"=w26:string, "Tabor Address"=w20:string)
  n196 = global write "SwitchGlobals.vi" "USB Switch"(w14) -> ()
  n197 = global write "PulserGlobals.vi" "Panametrics"(w13) -> ()
  n198 = global write "PulserGlobals.vi" "JSR VISA"(w9) -> ()
  n199 = global write "SwitchGlobals.vi" "Dual XDCR Settings"(w8) -> ()
  n200 = Unbundle By Name(w8) -> ("Scan Size"=w10:dbl[])
  n201 = Unbundle By Name(w8) -> ("XDCR Settings"=w7:T3[])
  n202 = Decrement(x=w4) -> (x-1=w3:u32)
  n203 = global write "SwitchGlobals.vi" "Full Scan Size"(w10) -> ()
  n204 = Index Array(array=w7, index=w3) -> (element=w6:T3)
  n205 = global write "PulserGlobals.vi" "Tabor"(w20) -> ()
  n206 = call "CreateDataFolders.vi"("Location In"="Location In", "Create Data Folder"="Create Data Folder", "Data Drive"=w26) -> ()  [unwired: 9 in]
  n207 = Unbundle By Name(w6) -> ("JSR Complete"=w5:T6, "UT340 Controls"=w1:T21)
  n208 = global write "PulserGlobals.vi" "JSR Settings"(w5) -> ()
  n209 = global write "PulserGlobals.vi" "UT340 Controls"(w1) -> ()
